vi "slow_control_2_06.vi"() -> ()   [LabVIEW 2018]
uses:
  <vilib>/DAQmx/read.llb/DAQmx Read (Analog 1D DBL NChan 1Samp).vi
  <vilib>/DAQmx/create/channels.llb/DAQmx Create Channel (AI-Voltage-Basic).vi
  <vilib>/DAQmx/create/channels.llb/DAQmx Create Channel (AI-Current-Basic).vi
  <vilib>/DAQmx/create/channels.llb/DAQmx Create Channel (AI-Temperature-RTD).vi
  <vilib>/DAQmx/miscellaneous.llb/DAQmx Fill In Error Info.vi
  <instrlib>/Lake Shore 335/Lake Shore 335.lvlib
  <instrlib>/CAEN PSM/CAEN PSM.lvlib
  <resource>/objmgr/daqmx.rc
panel:
  out "Channel Names":string[](array[string])
  out "Heater":dbl
  out "Coldhead":dbl
  out "Cycle number":i32
  in  "Cycles to execute":dbl=5.0 format="%#_13g"
  out "Moving average Det. P":dbl
  in  "N samples":i32=20
  in  "Allows tabs on \nfront panel":T1(tab)
  out "Valid example:":string
  in  "Specify which temperature sensors are\ninside the detector, separated with a comma.\nNumbers only, single commas, no empty strings!":string="10,11,12,13,14,15"
  in  "Anode ch.":enum16{"1", "2", "3", "4"}(ring)=enum."3"
  in  "CAEN unit selector":enum16{"CAEN 1", "CAEN 2"}(ring)
  in  "Multipliers":dbl[](array[numeric])=[1.0, 1.0, 1.0, 1.0, 1.0, 1.0, 1.0, 1.0]
  in  "Offsets\nsubtracted":dbl[](array[numeric])=[0.0, 0.0, 0.0, 0.0, 0.0, 0.0, 0.0, 0.0]
  in  "Channel Names (9207, ai8:15)":string[](array[string])=["i0", "i1", "i2", "i3", "i4", "i5", "i6", "i7"] caption="\"Other\""
  in  "Flow meter input:":T2(ring)=enum."v3"
  in  "Detector pressure input:":T2(ring)
  in  "Channel Names (9207, ai0:7)":string[](array[string])=["v0", "v1", "v2", "v3", "v4", "v5", "v6", "v7"] caption="\"Other\""
  in  "Multipliers":dbl[](array[numeric])=[0.2, 1.0, 1.0, 28.409091, 1.0, 1.0, 1.0, 1.0]
  in  "Offsets\nsubtracted":dbl[](array[numeric])=[0.002, 0.0, 0.0, 0.44376, 0.0, 0.0, 0.0, 0.0]
  in  "Voltage channels":tag[](array[tag])=["9207/ai0", "9207/ai1", "9207/ai2", "9207/ai3", "9207/ai4", "9207/ai5", "9207/ai6", "9207/ai7"]
  in  "COM-port CAEN 1":refnum<visa-resource-name>
  in  "COM-port CAEN 2":refnum<visa-resource-name>
  out "Temp B":dbl
  out "Temp A":dbl
  out "LakeShore readings 2":dbl[](array[numeric])
  in  "Run lakeshore?":bool
  in  "ID Query":bool=TRUE
  in  "COM-port LakeShore":refnum<visa-resource-name>
  in  "PID settings":cluster{"P":dbl, "I":dbl, "D":dbl}={"P"=50.0, "I"=20.0, "D"=120.0}
  in  "Setpoint (°C)":dbl=-100.0 format="%.1f"
  in  "Heater range":u16(ring) items=["Off", "Low (On)", "Medium", "High"]
  in  "Current channels":tag[](array[tag])=["9207/ai8", "9207/ai9", "9207/ai10", "9207/ai11", "9207/ai12", "9207/ai13", "9207/ai14", "9207/ai15"]
  in  "Channel Names (CAEN)":string[](array[string])=["PMT 1", "PMT 2", "Anode", "Cathode", "Top gate", "Bottom gate", "Other 1", "Other 2"]
  in  "RTD Type":i32(ring)=12481 items=["Pt3750"=12481, "Pt3851"=10071, "Pt3911"=12482, "Pt3916"=10069, "Pt3920"=10053, "Pt3928"=12483, "Custom"=10137]
  in  "Module 1 channels (slot 1)":tag[](array[tag])
  in  "Current Excitation Source":i32(ring)=10230 items=["Internal"=10200, "External"=10167, "None"=10230]
  in  "Resistance Configuration":i32(ring)=2 items=["2-Wire"=2, "3-Wire"=3, "4-Wire"=4]
  in  "R (T = 0°C):":dbl
  in  "B":dbl
  in  "A":dbl
  in  "C":dbl
  in  "Module 2 channels (slot 2)":tag[](array[tag])
  out "Array":i32[](array[numeric])
  out "9207 (V; A) Converted":dbl[](array[numeric])
  out "9216 #1 (°C)":dbl[](array[numeric])
  out "9216 #2 (°C)":dbl[](array[numeric])
  out "Readouts (V, mA)":dbl[](array[numeric]) format="%0.2f"
  out "Det.P input #":i32
  out "Flow input #":i32
  in  "T 20":bool
  in  "T 19":bool
  in  "T 18":bool
  in  "T 17":bool
  in  "T 16":bool
  in  "T 15":bool
  in  "Detector P":bool
  in  "Overpressure threshold":dbl
  in  "Underpressure threshold":dbl
  out "Comm. status":bool
  in  "High Temp threshold":dbl format="%#_13g"
  in  "Low Temp threshold":dbl format="%#_13g"
  in  "Ignore Initialization Errors":bool=TRUE caption="Ignore init. errors?"
  out "LakeShore status":bool
  out "NI mod1 (P) status":bool
  out "CAEN 1 status":bool
  out "CAEN 2 status":bool
  out "Initialization status":bool
  in  "Temperature channel selector":u16(ring)=10 items=["10"=10, "11"=11, "12"=12, "13"=13, "14"=14, "15"=15, "Average"=666]
  out "Heater power (%)":cluster{timestamp[], dbl[]}[](graph)
  out "Flow (SLPM)":cluster{timestamp[], dbl[]}[](graph)
  out "9207 (ai0:7)":cluster{timestamp[], dbl[]}[](graph)
  out "Phase Diagram":cluster{"X":dbl, "Y":dbl}[](graph)
  out "Temperature":cluster{timestamp[], dbl[]}[](graph)
  in  "N samples":i32=30
  out "Average Flow (SLPM)":dbl caption="Average Flow (SLPM), of"
  in  "Pause?":bool
  out "Integrated Flow (SL)":dbl
  in  "Reset?":bool
  out "LakeShore readings":dbl[](array[numeric])
  in  "Temperature Channel Selector":u16(ring) items=["10"=10, "11"=11, "12"=12, "13"=13, "14"=14, "15"=15]
  out "Historical Large Phase Diagram":cluster{dbl[], dbl[]}[](graph)
  out "Large Phase Diagram":cluster{"X":dbl, "Y":dbl}[](graph)
  in  "Temperature Channel Selector":u16(ring)=666 items=["10"=10, "11"=11, "12"=12, "13"=13, "14"=14, "15"=15, "Average"=666]
  in  "Scale.Range:Minimum 8":dbl
  in  "Scale.Range:Maximum 8":dbl=4000.0
  in  "Scale.Range:Minimum 7":dbl
  in  "Scale.Range:Maximum 7":dbl=4000.0
  in  "Scale.Range:Minimum 6":dbl=-3000.0
  in  "Scale.Range:Maximum 6":dbl
  in  "Scale.Range:Minimum 5":dbl
  in  "Scale.Range:Maximum 5":dbl=3000.0
  in  "Scale.Range:Minimum 4":dbl=-5000.0
  in  "Scale.Range:Maximum 4":dbl
  in  "Scale.Range:Maximum 3":dbl=4000.0
  in  "Scale.Range:Minimum 3":dbl
  in  "Scale.Range:Maximum 2":dbl=1000.0
  in  "Scale.Range:Minimum 2":dbl
  out "CAEN 1.1":dbl(knob) scale=0.0..1000.0
  out "CAEN 1.1":string
  in  "Scale.Range:Maximum":dbl=1000.0
  in  "Scale.Range:Minimum":dbl
  out "CAEN 2.3 2":string
  out "CAEN 2.2 2":string
  out "Channel Names":string[](array[string])
  out "CAEN 2.3":dbl(knob) scale=0.0..4000.0
  out "CAEN 2.2":dbl(knob) scale=0.0..4000.0
  out "CAEN 2.1":string
  out "CAEN 2.0":string
  out "CAEN 1.3":string
  out "CAEN 1.2":string
  out "CAEN 1.0":string
  out "Channel Names":string[](array[string])
  in  "Set to zero":bool
  out "CAEN 2.1":dbl(knob)
  out "CAEN 2.0":dbl(knob) scale=0.0..3000.0
  in  "Apply Voltage":bool
  in  "VSet (V)":dbl[](array[numeric])
  in  "IMax (uA)":dbl[](array[numeric])
  in  "VMax (V)":dbl[](array[numeric])
  out "CAEN 1.3":dbl(knob)
  out "CAEN 1.2":dbl(knob) scale=0.0..4000.0
  out "CAEN 1.0":dbl(knob) scale=0.0..1000.0
  out "Vmon (V)":dbl[](array[numeric])
  out "IMon (uA)":dbl[](array[numeric])
  in  "Read V every N cycles":i16=120
  in  "Reset anode":bool
  in  "Kill every Y minutes":i32=10
  in  "Keep off for X seconds":i32=10
  out "?":bool
  out "Killed":bool
  out "Restarted":bool
  out "Anode times":dbl[](array[numeric]) format="%_12f"
  out "Anode times 2":timestamp[](array[timestamp])
  in  "Kill voltage":bool
  in  "stop":bool
  out "Voltages":dbl[](array[numeric])
  out "Started up?":bool
  out "TOBA appended":dbl[][](array[numeric])
  in  "Read T every N cycles":i32=2
  out "Time until next cycle":dbl format="%.3g"
  in  "Time per cycle (s)":i32=2 caption="Time Target (s)"
  # "<- Proof of concept for New/Old T + New P"
  # "NI 9216 Temperature settings"
  # "CAEN settings"
  # "NI 9207 Voltage settings"
  # "If RTD type is custom,\nspecify the Callendar-\nVan Dusen parameters"
  # "Anode connected to:"
  # "Channel:"
  # "Lakeshore settings"
  # "NI 9207 Current settings"
  # "Connection settings"
  # "Gain (P) (XX.X)"
  # "Reset (I) (XX.X)"
  # "Rate (D) (X.X%)"
  # "Move to Quick Temp tab ^"
  # "Alarm indicators"
  # "Thresholds"
  # "Alarm conditions"
  # "Data"
  # "Time of last reset"
  # "Scale:"
  # "to"
  # "to"
  # "Scale:"
  # "Time of last reactivation"
  # "Settings"
  # "to"
  # "Scale:"
  # "to"
  # "Scale:"
  # "Scale:"
  # "to"
  # "Scale:"
  # "to"
  # "Scale:"
  # "to"
  # "to"
  # "Scale:"
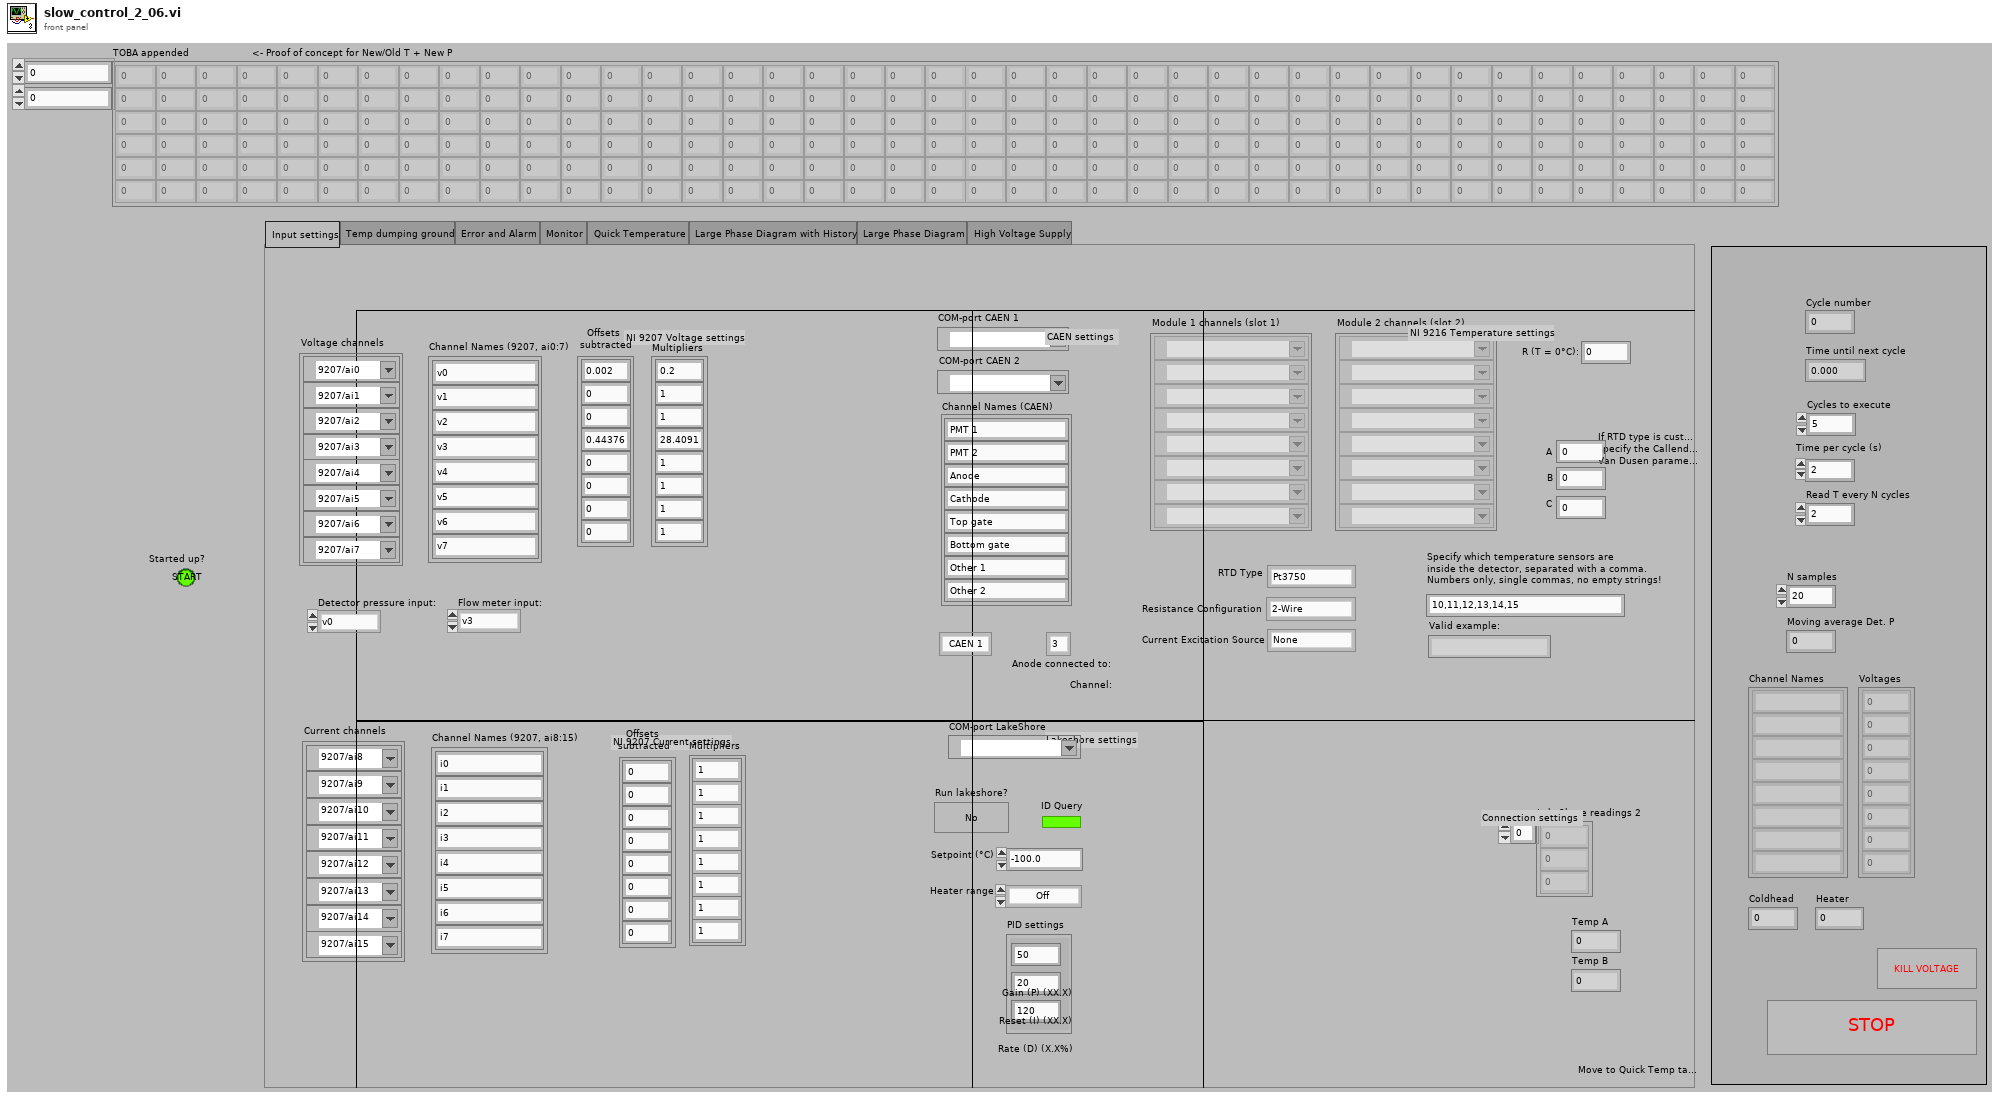
[diagram p1: front panel]
types:
  T1 = enum32{"Input settings", "Temp dumping ground", "Error and Alarm", "Monitor", "Quick Temperature", "Large Phase Diagram with History", "Large Phase Diagram", "High Voltage Supply"}
  T2 = enum16{"v0", "v1", "v2", "v3", "v4", "v5", "v6", "v7"}
  T3 = cluster{"Baud Rate":u32, "Parity":u16, "Data Bits":u16, "Stop Bits":u16, "Flow Control":u16}
  T4 = cluster{"VISA resource name out":refnum<visa-resource-name>, "error out":errorcluster}
  T5 = cluster{"task out":refnum<k21>, "error out":errorcluster}
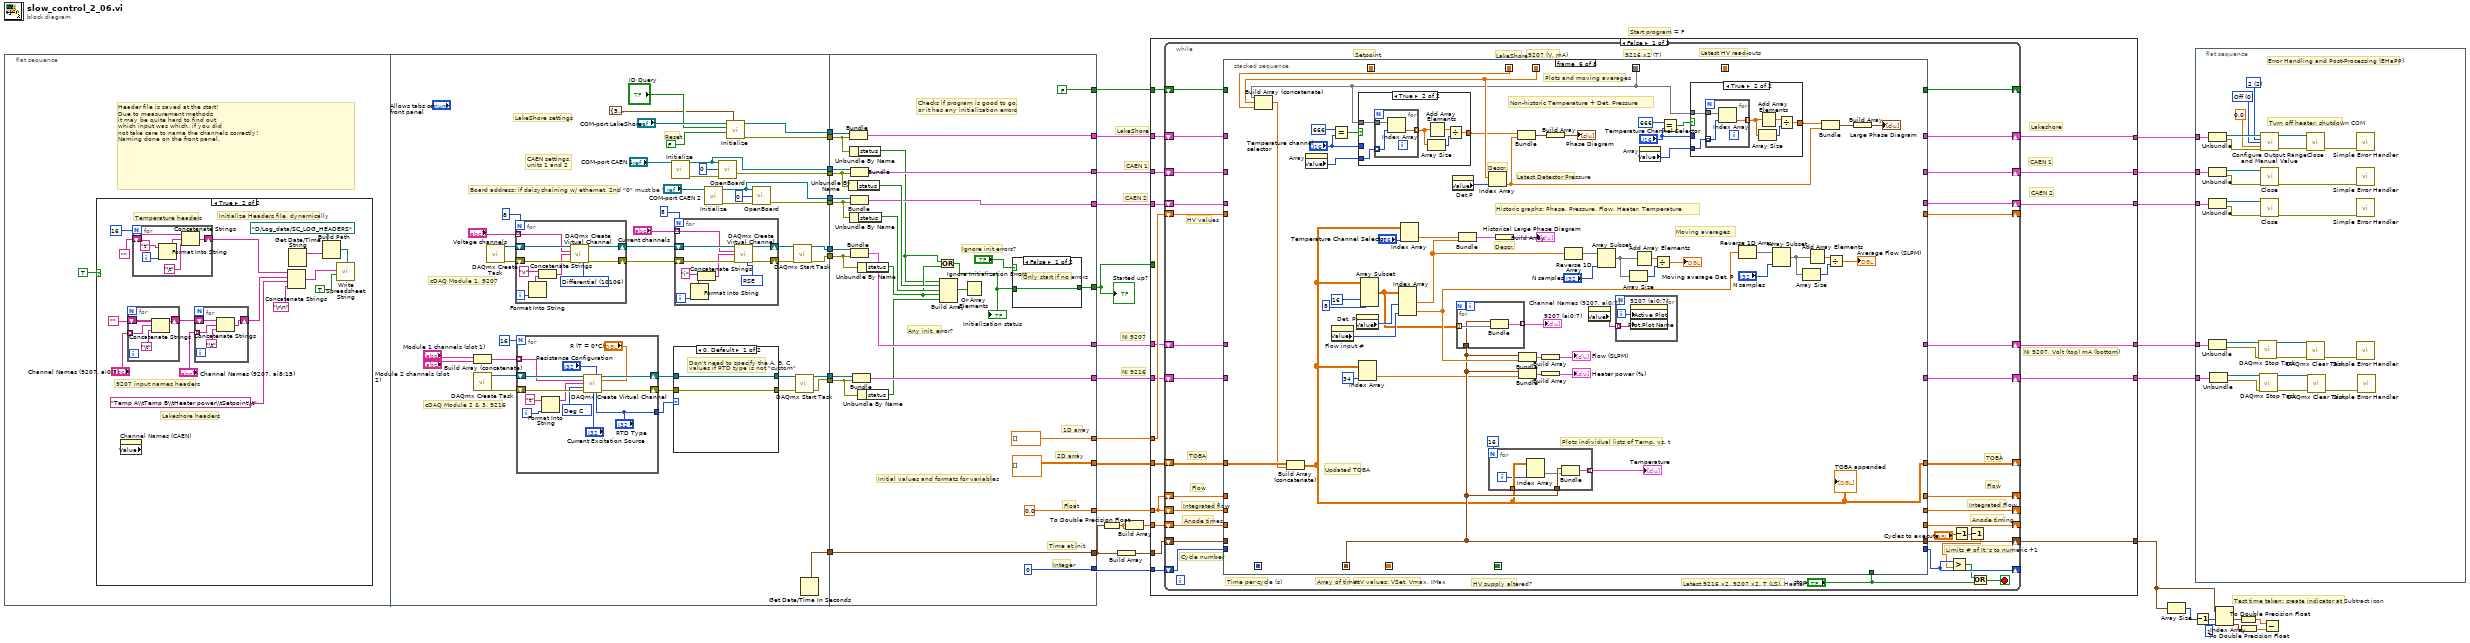
[diagram p0: block diagram]
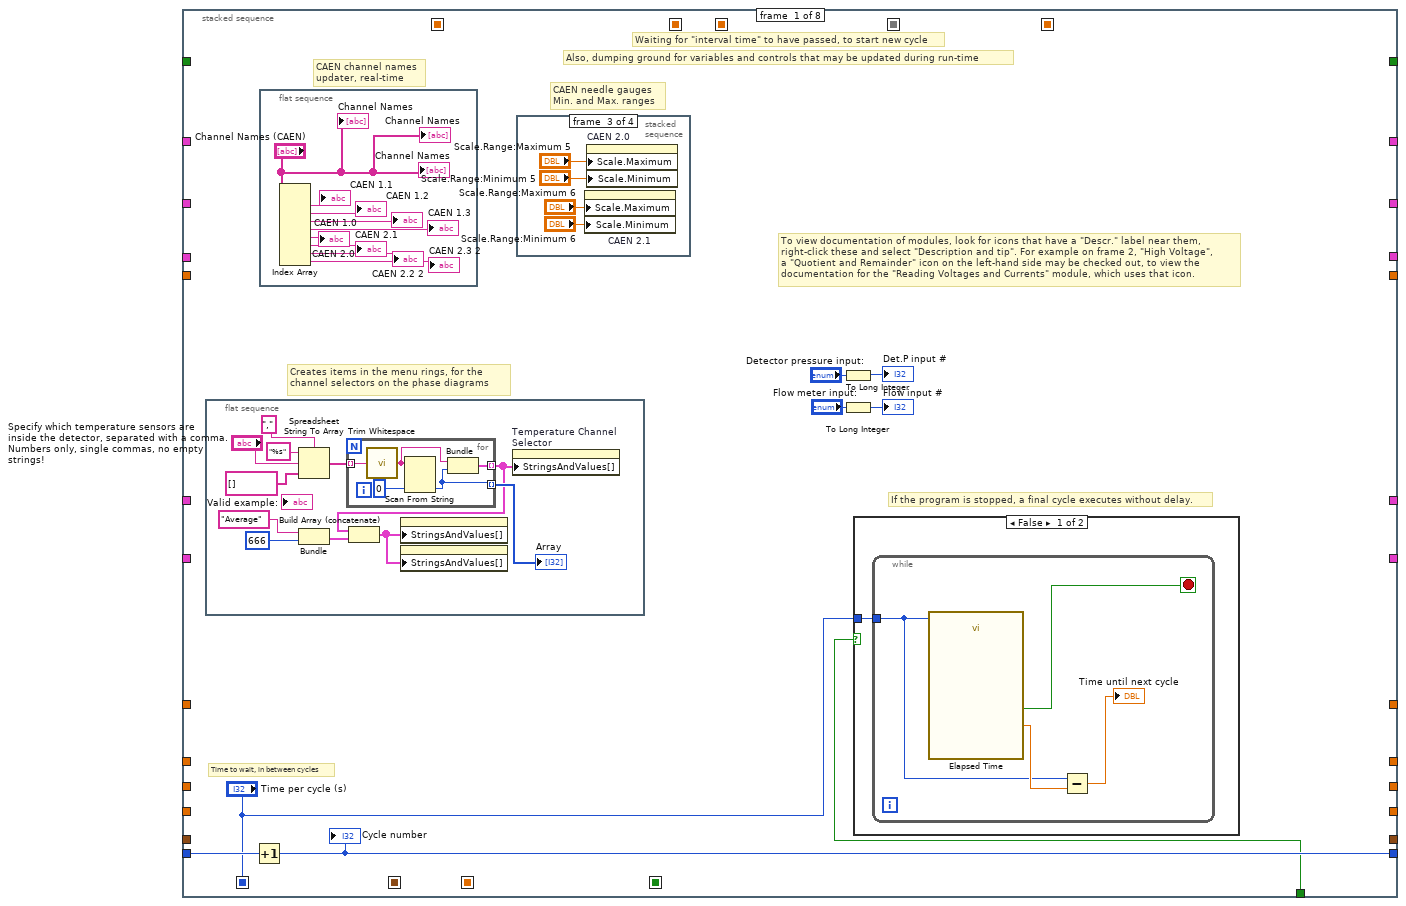
[diagram p2: hidden frame]
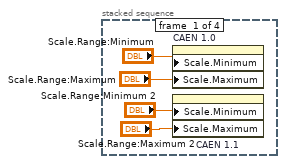
[diagram p3: hidden frame]
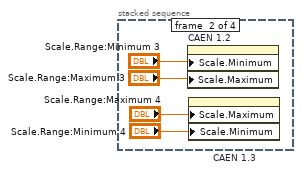
[diagram p4: hidden frame]
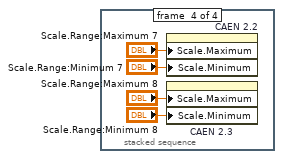
[diagram p5: hidden frame]
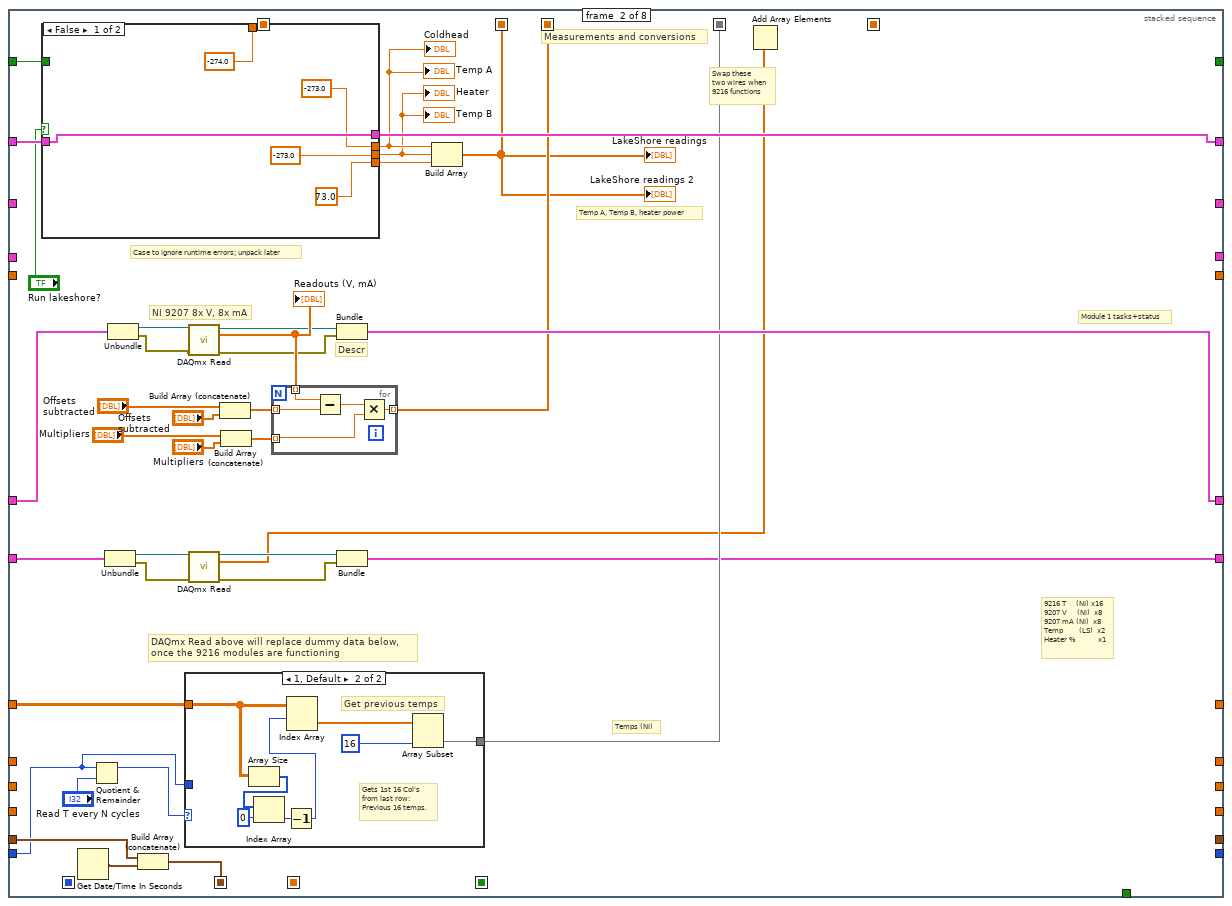
[diagram p7: hidden frame]
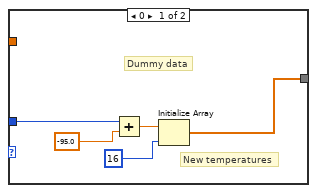
[diagram p8: hidden frame]
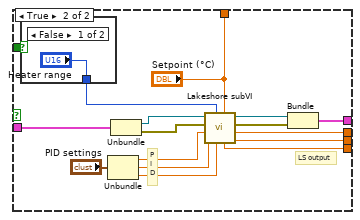
[diagram p9: hidden frame]
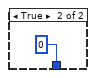
[diagram p10: hidden frame]
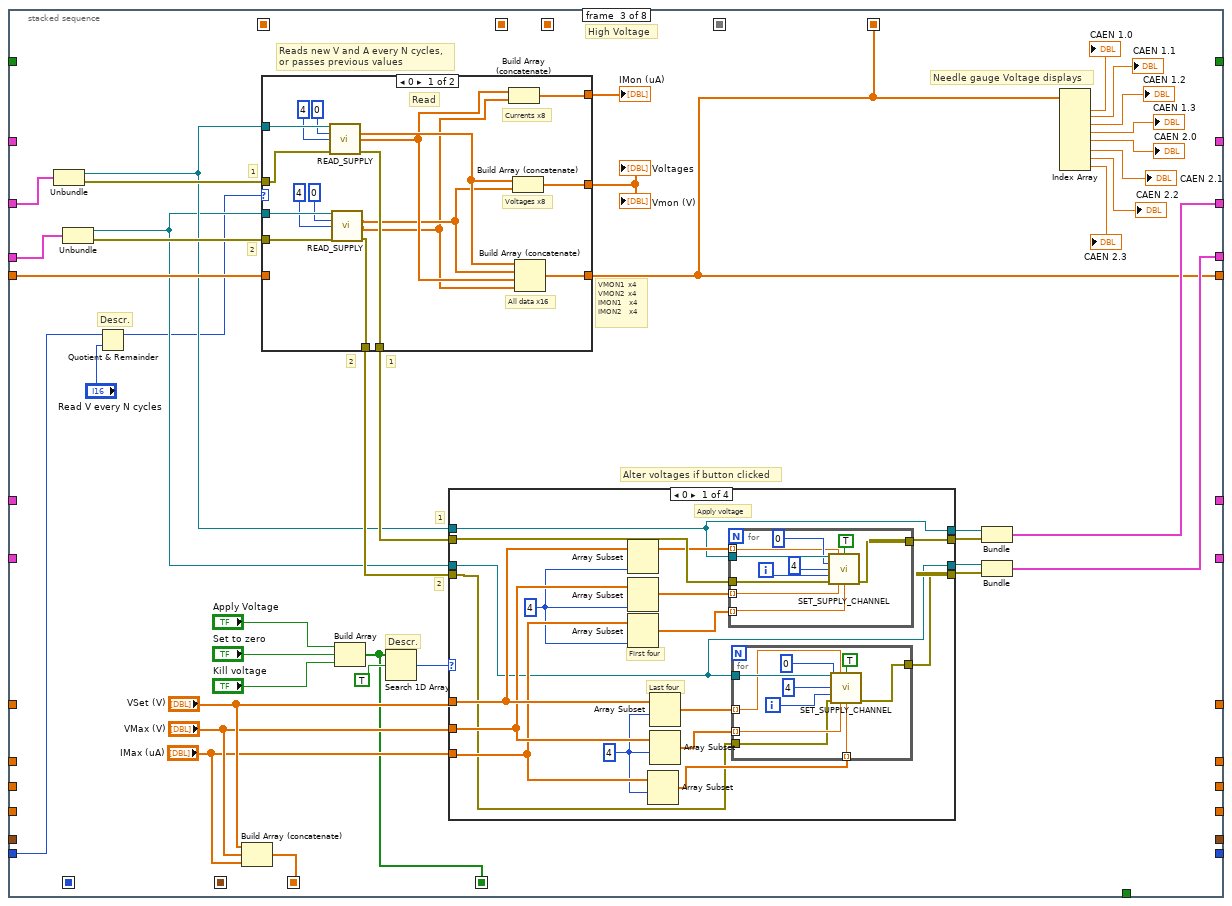
[diagram p11: hidden frame]
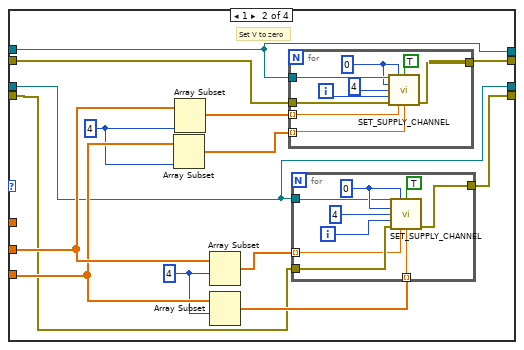
[diagram p12: hidden frame]
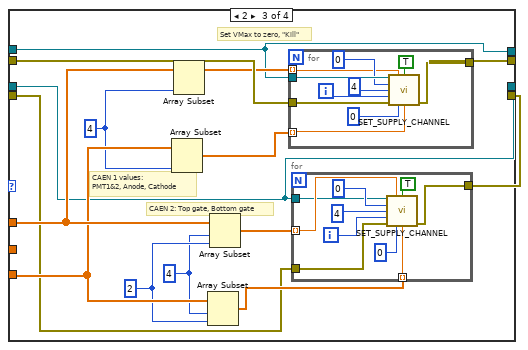
[diagram p13: hidden frame]
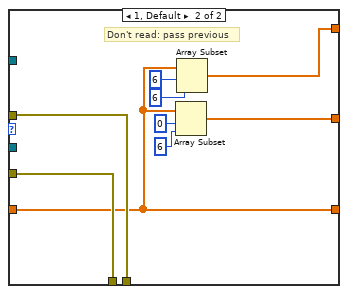
[diagram p15: hidden frame]
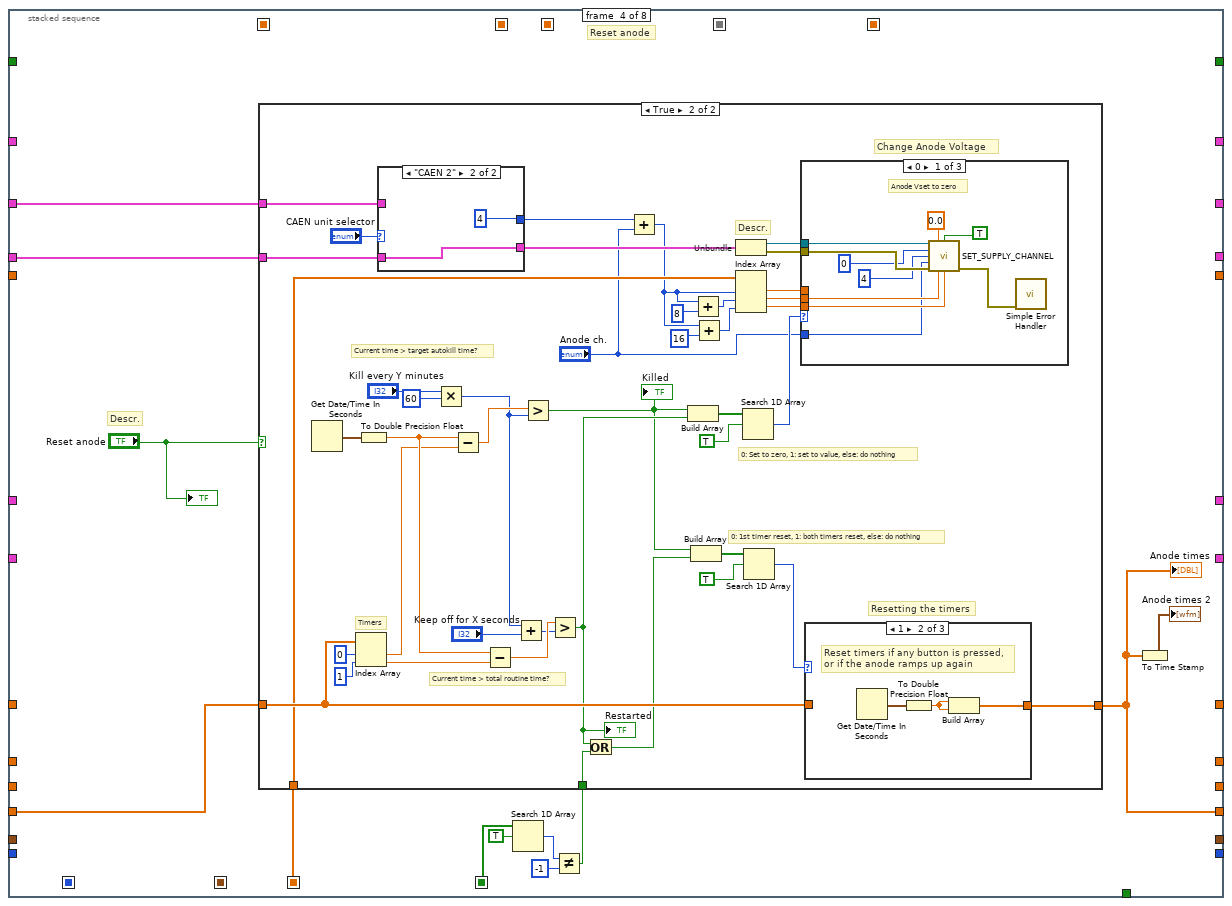
[diagram p16: hidden frame]
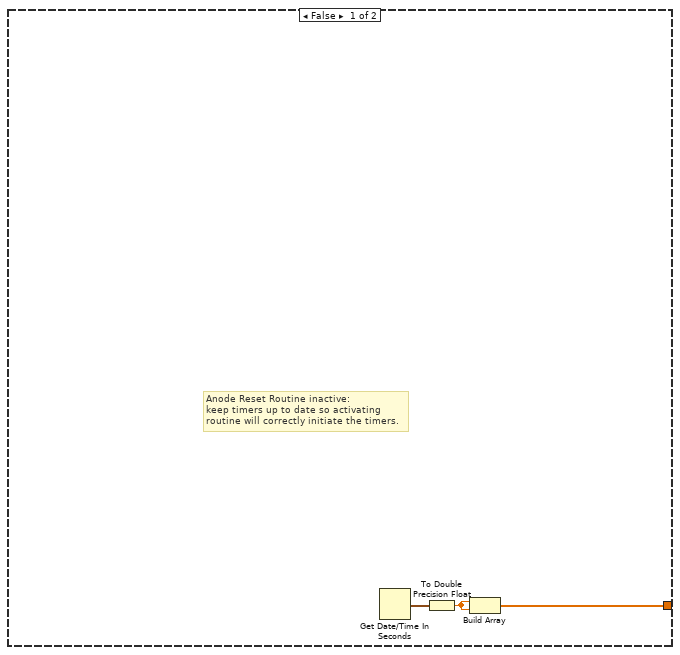
[diagram p17: hidden frame]
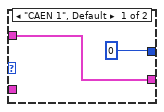
[diagram p18: hidden frame]
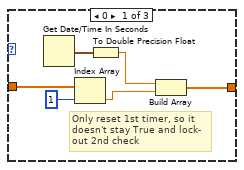
[diagram p19: hidden frame]
diagram:
  # "NI 9216"
  # "Test time taken: create indicator at Subtract icon"
  # "NI 9207"
  # "Start program = F"
  # "CAEN 2"
  # "CAEN 1"
  # "LakeShore"
  n1 = flat-sequence {
    tunnel: [w108] -> w39
    tunnel: [w107] -> w38
    tunnel: [w95] -> w37
    tunnel: [w104] -> w36
    tunnel: [w85] -> w35
    tunnel: [w103] -> w30
    tunnel: [w99] -> w22
    tunnel: [w98] -> w21
    tunnel: [w86] -> w12
    tunnel: [w80] -> w4
    tunnel: [w79] -> w3
    tunnel: w39 -> [w180]
    tunnel: w38 -> [w179]
    tunnel: w37 -> [w177]
    tunnel: w36 -> [w176]
    tunnel: w35 -> [w166]
    tunnel: [w181] -> w19
    tunnel: [0.0] -> w18
    tunnel: [dbl[] []] -> w34
    tunnel: [dbl[][] []] -> w5
    tunnel: [0] -> w33
    tunnel: [w178] -> w32
    tunnel: [w175] -> w31
    tunnel: [w174] -> w17
    tunnel: w30 -> [w174]
    tunnel: w22 -> [w172]
    tunnel: w21 -> [w171]
    tunnel: [w170] -> w20
    tunnel: [FALSE] -> w13
    tunnel: w12 -> [w167]
    tunnel: [w165] -> w11
    tunnel: w4 -> [w157]
    tunnel: w3 -> [w156]
    tunnel: [w155] -> w2
    frame #0 {
      # "Header file is saved at the start!\nDue to measurement methods\nit may be quite hard to find out\nwhich input was which, if you did\nnot take care to name the channels correctly!\nNaming done on the front panel."
      n2 = case shown="True" TRUE {
        frame False {
        }
        frame True {
          # "Lakeshore headers"
          # "9207 input names headers"
          # "Temperature headers"
          # "Initialize Headers file, dynamically"
          n3 = property on="Channel Names (CAEN)" class="Arr (strict)" props=["Value"]() -> ()  [unwired: 2 in, 3 out]
          n4 = for {
            shift-right: [w62] -> w44
            shift-left: "" -> [w63]
            tunnel: "Channel Names (9207, ai0:7)" -> [w60] mode=indexing
            n5 = Concatenate Strings(w63, w60, "\t") -> (w62:string)
          }
          n6 = for {
            N: 16 -> [_]
            shift-right: [w64] -> w47
            shift-left: "" -> [w65]
            i -> [w69]
            n7 = Format Into String(initial string="t", w69) -> (resulting string=w67:string)  [unwired: 2 in, 1 out]
            n8 = Concatenate Strings(w65, w67, "\t") -> (w64:string)
          }
          n9 = for {
            shift-right: [w57] -> w43
            shift-left: w44 -> [w59]
            tunnel: "Channel Names (9207, ai8:15)" -> [w56] mode=indexing
            n10 = Concatenate Strings(w59, w56, "\t") -> (w57:string)
          }
          n11 = Concatenate Strings(w47, w43, "Temp A\\tTemp B\\tHeater power\\tSetpoint\\t", "\r\n") -> (w46:string)
          n12 = Get Date/Time String() -> (date string=w50:string)  [unwired: 3 in, 1 out]
          n13 = Build Path(base path=path "D:/Log_data/SC_LOG_HEADERS" ("file path (dialog if empty)"), name or relative path=w50) -> (appended path=w51:path)
          n14 = call <vilib>:"Write Spreadsheet String.vi"("append to file? (new file:F)"=TRUE, "spreadsheet string"=w46, "file path (dialog if empty)"=w51) -> ()  [unwired: 7 in, 2 out]
        }
      }
    }
    frame #1 {
      # "cDAQ Module 2 & 3, 9216"
      # "cDAQ Module 1, 9207"
      # "Board address: if daisychaining w/ ethernet, 2nd \"0\" must be \"1\""
      # "CAEN settings,\nunits 1 and 2"
      # "Reset"
      # "LakeShore settings"
      n15 = call <vilib>:"DAQmx Create Task.vi"() -> ("task out"=w78:refnum<k21>, "error out"=w81:errorcluster)  [unwired: 14 in]
      n16 = Build Array (concatenate)("Module 1 channels (slot 1)", "Module 2 channels (slot 2)") -> (w75:tag[])
      n17 = call <vilib>:"DAQmx Create Task.vi"() -> ("task out"=w94:refnum<k21>, "error out"=w93:errorcluster)  [unwired: 14 in]
      n18 = for {
        N: 8 -> [_]
        shift-right: [w149] -> w90
        shift-left: w94 -> [w148]
        shift-right: [w150] -> w89
        shift-left: w93 -> [w146]
        tunnel: "Voltage channels" -> [w147] mode=indexing
        i -> [w152]
        w144 = 10106 items=["Default"=-1, "RSE"=10083, "NRSE"=10078, "Differential"=10106, "Pseudodifferential"=12529] ("input terminal configuration")
        n19 = Format Into String(w152) -> (resulting string=w151:string)  [unwired: 3 in, 1 out]
        n20 = Concatenate Strings("v" ("string"), w151) -> (w145:string)
        n21 = call-poly <vilib>:"DAQmx Create Virtual Channel.vi"("task in"=w148, "input terminal configuration"=w144, "physical channels"=w147, "name to assign"=w145, "error in"=w146) -> ("task out"=w149:refnum<k21>, "error out"=w150:errorcluster)  [unwired: 9 in]
      }
      n22 = for {
        N: 16 -> [_]
        shift-right: [w130] -> w74
        shift-left: w78 -> [w133]
        shift-right: [w131] -> w73
        shift-left: w81 -> [w132]
        tunnel: w75 -> [w129] mode=indexing
        tunnel: ["RTD Type"] -> w70
        i -> [w127]
        w124 = 10143 items=["Deg C"=10143, "Deg F"=10144, "Kelvins"=10325, "Deg R"=10145, "From Custom Scale"=10065] ("units")
        n23 = Format Into String(initial string="t", w127) -> (resulting string=w126:string)  [unwired: 2 in, 1 out]
        n24 = call-poly <vilib>:"DAQmx Create Virtual Channel.vi"("task in"=w133, "resistance configuration"="Resistance Configuration", "physical channels"=w129, "r0"="R (T = 0°C):", "name to assign"=w126, "units"=w124, "error in"=w132, "current excitation source"="Current Excitation Source", "rtd type"="RTD Type") -> ("task out"=w130:refnum<k21>, "error out"=w131:errorcluster)  [unwired: 5 in]
      }
      n25 = call <instrlib>:"Initialize.vi"("VISA resource name"="COM-port CAEN 1") -> ("error out"=w105:errorcluster, "VISA resource name out"=w95:refnum<visa-resource-name>)  [unwired: 9 in]
      n26 = case shown="0, Default" w70 {
        tunnel: w74 -> [w113 w117]
        tunnel: w73 -> [w112 w116]
        tunnel: [w113 w115] -> w72
        tunnel: [w112 w114] -> w71
        frame 0, Default {
          # "Don't need to specify the A, B, C\nvalues if RTD type is not \"custom\""
        }
        frame 10137 {
          # "RTD type =  \"custom\""
          n27 = property class="DAQmx Channel"(reference=w117, error in=w116, "AI.RTD.A"="A", "AI.RTD.B"="B", "AI.RTD.C"="C") -> (reference out=w115:refnum<k21>, error out=w114:errorcluster)
        }
      }
      n28 = for {
        N: 8 -> [_]
        shift-right: [w135] -> w87
        shift-left: w90 -> [w142]
        shift-right: [w134] -> w88
        shift-left: w89 -> [w141]
        tunnel: "Current channels" -> [w140] mode=indexing
        i -> [w139]
        w143 = 10083 items=["default"=-1, "RSE"=10083, "NRSE"=10078, "Differential"=10106, "Pseudodifferential"=12529] ("input terminal configuration")
        n29 = Format Into String(w139) -> (resulting string=w137:string)  [unwired: 3 in, 1 out]
        n30 = Concatenate Strings("i", w137) -> (w136:string)
        n31 = call-poly <vilib>:"DAQmx Create Virtual Channel.vi"("task in"=w142, "input terminal configuration"=w143, "physical channels"=w140, "name to assign"=w136, "error in"=w141) -> ("task out"=w135:refnum<k21>, "error out"=w134:errorcluster)  [unwired: 9 in]
      }
      n32 = call <instrlib>:"Initialize.vi"("VISA resource name"="COM-port CAEN 2") -> ("error out"=w100:errorcluster, "VISA resource name out"=w99:refnum<visa-resource-name>)  [unwired: 9 in]
      n33 = call <instrlib>:"OpenBoard.vi"("error in (no error)"=w105, "Board Address"=0, "VISA resource name"=w95) -> ("error out"=w104:errorcluster)  [unwired: 7 in, 1 out]
      n34 = call <instrlib>:"Initialize.vi"("Serial Configuration"=T3 {"Baud Rate"=57600, "Parity"=1, "Data Bits"=7, "Stop Bits"=10, "Flow Control"=0}, "Reset (True)"=FALSE ("Reset (LakeShore)"), "ID Query (True)"="ID Query", "VISA resource name"="COM-port LakeShore") -> ("error out"=w107:errorcluster, "VISA resource name out"=w108:refnum<visa-resource-name>)  [unwired: 6 in]
      n35 = call <instrlib>:"OpenBoard.vi"("error in (no error)"=w100, "Board Address"=u8 0, "VISA resource name"=w99) -> ("error out"=w98:errorcluster)  [unwired: 7 in, 1 out]
      n36 = call <vilib>:"DAQmx Start Task.vi"("task/channels in"=w87, "error in"=w88) -> ("task out"=w86:refnum<k21>, "error out"=w85:errorcluster)  [unwired: 12 in]
      n37 = call <vilib>:"DAQmx Start Task.vi"("task/channels in"=w72, "error in"=w71) -> ("task out"=w80:refnum<k21>, "error out"=w79:errorcluster)  [unwired: 12 in]
      n38 = Get Date/Time In Seconds() -> (seconds since 1Jan1904=w103:timestamp)
    }
    frame #2 {
      # "Initial values and formats for variables"
      # "Time at init."
      # "Integer"
      # "2D array"
      # "1D array"
      # "Float"
      # "Checks if program is good to go,\nor it has any initialization errors"
      # "Ignore init errors?"
      # "Any init. error?"
      n39 = Unbundle By Name(w176) -> ("status"=w182:bool)
      n40 = Unbundle By Name(w179) -> ("status"=w159:bool)
      n41 = Bundle("VISA resource name out"=w180, "error out"=w179) -> (w178:T4)  [unwired: 1 in]
      n42 = Unbundle By Name(w171) -> ("status"=w173:bool)
      n43 = Bundle("VISA resource name out"=w172, "error out"=w171) -> (w170:T4)  [unwired: 1 in]
      n44 = Bundle("task out"=w167, "error out"=w166) -> (w165:T5)  [unwired: 1 in]
      n45 = Bundle("VISA resource name out"=w177, "error out"=w176) -> (w175:T4)  [unwired: 1 in]
      n46 = Bundle("task out"=w157, "error out"=w156) -> (w155:T5)  [unwired: 1 in]
      n47 = Unbundle By Name(w166) -> ("status"=w160:bool)
      n48 = Unbundle By Name(w156) -> ("status"=w154:bool)
      n49 = Or(x=w159, y=w160) -> (x .or. y?=w158:bool)
      "Initialization status" <- w158
      n50 = Build Array(w159, w182, w160, w173, w154) -> (w183:bool[])
      n51 = Or Array Elements(Boolean array=w183) -> ()  [unwired: 1 out]
      n52 = case shown="False" "Ignore Initialization Errors" {
        tunnel: [w184 FALSE] -> w181
        tunnel: w158 -> [w184 _]
        frame False {
          # "Only start if no errors"
        }
        frame True {
          # "Always start program"
        }
      }
    }
  }
  n53 = To Double Precision Float(number=w17) -> (double precision float=w16:dbl)
  n54 = Build Array(w17) -> (w29:timestamp[])
  n55 = Build Array(w16, w16) -> (w15:dbl[])
  n56 = case shown="False" w19 {
    selector: w19 -> [_ w784]
    tunnel: [_ w784] -> _
    tunnel: w34 -> [w196 _]
    tunnel: w33 -> [w203 _]
    tunnel: w5 -> [w202 _]
    tunnel: w32 -> [w197 w782]
    tunnel: w31 -> [w199 w781]
    tunnel: w29 -> [w201 _]
    tunnel: [w200 timestamp[] []] -> w25
    tunnel: w20 -> [w198 w780]
    tunnel: w18 -> [w192 _]
    tunnel: w15 -> [w195 _]
    tunnel: [w194 w782] -> w14
    tunnel: w13 -> [w193 _]
    tunnel: w11 -> [w191 w779]
    tunnel: [w190 w781] -> w10
    tunnel: [w189 w780] -> w9
    tunnel: [w188 w779] -> w8
    tunnel: w2 -> [w187 w778]
    tunnel: [w186 w778] -> w1
    frame False {
      # "NI 9207, Volt (top) mA (bottom)"
      # "CAEN 2"
      # "CAEN 1"
      # "Lakeshore"
      n57 = while {
        shift-right: [w230] -> _
        shift-left: w203 -> [w235]
        shift-right: [w232] -> _
        shift-left: w202 -> [w221]
        shift-right: [w222] -> w200
        shift-left: w201 -> [w231]
        shift-right: [w224] -> w190
        shift-left: w199 -> [w216]
        shift-right: [w226] -> _
        shift-left: w196 -> [w229]
        shift-right: [w223] -> w189
        shift-left: w198 -> [w228]
        shift-right: [w225] -> w194
        shift-left: w197 -> [w227]
        shift-right: [w209] -> _
        shift-left: w192 -> [w218]
        shift-right: [w208] -> _
        shift-left: w192 -> [w219]
        shift-right: [w215] -> _
        shift-left: w195 -> [w217]
        shift-right: [w213] -> _
        shift-left: w193 -> [w214]
        shift-right: [w211] -> w188
        shift-left: w191 -> [w212]
        shift-right: [w206] -> w186
        shift-left: w187 -> [w207]
        stop <- w233 stop-if-true
        # "LakeShore"
        # "9216 x2 (T)"
        # "9207 (V, mA)"
        # "HV supply altered?"
        # "Setpoint"
        # "Anode timing"
        # "Anode times"
        # "Integrated flow"
        # "Flow"
        # "Flow"
        # "Integrated Flow"
        # "TOBA"
        # "Array of times"
        # "Latest HV read-outs"
        # "Time per cycle (s)"
        # "Cycle number"
        # "HV values: VSet, Vmax, IMax"
        # "HV values"
        # "TOBA"
        # "Latest 9216 x2, 9207 x2, T (LS), Heater% (LS)"
        # "Limits # of It.'s to numeric +1"
        n58 = stacked-sequence {
          seq-local: [_ _ w378 _ _ _ _ _] -> [_ _ _ w550 _ _ _ _]
          seq-local: ["Time per cycle (s)" _ _ _ _ _ _ _] -> [_ _ _ _ _ _ w755 _]
          seq-local: [_ _ w369 _ _ _ _ _] -> [_ _ _ _ _ _ w754 _]
          seq-local: [_ w322 _ _ _ _ _ _] -> [_ _ _ _ w640 w655 _ _]
          seq-local: [_ _ w372 _ _ _ _ _] -> [_ _ _ w553 _ _ _ _]
          seq-local: [_ w315 _ _ _ _ _ _] -> [_ _ _ _ _ _ w758 _]
          seq-local: [_ w310 _ _ _ _ _ _] -> [_ _ _ _ w633 w679 w742 _]
          seq-local: [_ w309 _ _ _ _ _ _] -> [_ _ _ _ w634 w669 w743 _]
          seq-local: [_ w297 _ _ _ _ _ _] -> [_ _ _ _ _ w677 w741 _]
          tunnel: [w242 _ _ _ _ _ _ _] -> w230
          tunnel: "stop" -> [w241 _ _ _ _ _ _ _]
          tunnel: w235 -> [w243 w311 w400 _ _ _ _ _]
          tunnel: w221 -> [_ w312 _ _ _ w681 _ _]
          tunnel: [_ _ _ _ _ w653 _ _] -> w232
          tunnel: w231 -> [_ w324 _ _ _ _ _ _]
          tunnel: w216 -> [_ _ w407 w551 _ _ _ w777]
          tunnel: w229 -> [_ _ w405 _ _ _ _ _]
          tunnel: w228 -> [_ _ w404 w542 _ _ _ w776]
          tunnel: w227 -> [_ w325 _ _ _ _ _ w775]
          tunnel: [_ w326 _ _ _ _ _ _] -> w225
          tunnel: [_ _ w369 _ _ _ _ _] -> w226
          tunnel: [_ _ w386 _ _ _ _ _] -> w224
          tunnel: [_ _ w383 _ _ _ _ _] -> w223
          tunnel: [_ _ _ _ _ w655 _ _] -> w222
          tunnel: w218 -> [_ _ _ _ w637 _ _ _]
          tunnel: w219 -> [_ _ _ _ w639 _ _ _]
          tunnel: w217 -> [_ _ _ w552 _ _ _ _]
          tunnel: [_ _ _ w546 _ _ _ _] -> w215
          tunnel: w214 -> [_ w318 _ _ _ _ _ _]
          tunnel: [_ _ _ _ _ _ _ FALSE] -> w213
          tunnel: w212 -> [_ w317 _ _ _ _ _ w773]
          tunnel: [_ w313 _ _ _ _ _ _] -> w211
          tunnel: [_ _ _ _ w636 _ _ _] -> w209
          tunnel: [_ _ _ _ w635 _ _ _] -> w208
          tunnel: w207 -> [_ w296 _ _ _ _ _ w759]
          tunnel: [_ w291 _ _ _ _ _ _] -> w206
          frame #0 {
            # "Creates items in the menu rings, for the channel selectors on the phase diagrams"
            # "Also, dumping ground for variables and controls that may be updated during run-time"
            # "CAEN needle gauges\nMin. and Max. ranges"
            # "CAEN channel names\nupdater, real-time"
            # "To view documentation of modules, look for icons that have a \"Descr.\" label near them,\nright-click these and select \"Description and tip\". For example on frame 2, \"High Voltage\",\na \"Quotient and Remainder\" icon on the left-hand side may be checked out, to view the\ndocumentation for the \"Reading Voltages and Currents\" module, which uses that icon."
            # "Time to wait, in between cycles"
            # "If the program is stopped, a final cycle executes without delay."
            # "Waiting for \"interval time\" to have passed, to start new cycle"
            n59 = flat-sequence {
              frame #0 {
                n60 = Spreadsheet String To Array(delimiter (Tab)=",", format string="%s", spreadsheet string="Specify which temperature sensors are\ninside the detector, separated with a comma.\nNumbers only, single commas, no empty strings!", array type (2D Dbl)=string[] []) -> (array=w250:string[])
                n61 = Bundle("Average", 666) -> (w247:cluster{string, i32})  [unwired: 1 in]
                n62 = for {
                  tunnel: w250 -> [w259] mode=indexing
                  tunnel: [w256] -> w244 mode=indexing
                  tunnel: [w255] -> w246 mode=indexing
                  n63 = call <vilib>:"Trim Whitespace.vi"("string"=w259) -> ("trimmed string"=w257:string)  [unwired: 1 in]
                  n64 = Scan From String(input string=w257, default 1=0) -> (output 1=w255:i32)  [unwired: 3 in, 3 out]
                  n65 = Bundle("trimmed string"=w257, w255) -> (w256:cluster{"trimmed string":string, i32})  [unwired: 1 in]
                }
                "Array" <- w246
                n66 = Build Array (concatenate)(w244, w247) -> (w245:cluster{"trimmed string":string, i32}[])
                n67 = property on="Temperature channel selector" class="Ring (strict)"("StringsAndValues[]"=w245) -> ()  [unwired: 2 in, 2 out]
                n68 = property on="Temperature Channel Selector" class="Ring (strict)"("StringsAndValues[]"=w245) -> ()  [unwired: 2 in, 2 out]
                n69 = property on="Temperature Channel Selector" class="Ring (strict)"("StringsAndValues[]"=w244) -> ()  [unwired: 2 in, 2 out]
              }
            }
            n70 = Increment(x=w243) -> (x+1=w242:i32)
            "Cycle number" <- w242
            n71 = flat-sequence {
              frame #0 {
                n72 = Index Array(array="Channel Names (CAEN)") -> (element #1=→"CAEN 1.0":string, element #2=→"CAEN 1.1":string, element #3=→"CAEN 1.2":string, element #4=→"CAEN 1.3":string, element #5=→"CAEN 2.0":string, element #6=→"CAEN 2.1":string, element #7=→"CAEN 2.2 2":string, element #8=→"CAEN 2.3 2":string)  [unwired: 8 in]
                "Channel Names" <- "Channel Names (CAEN)"
                "Channel Names" <- "Channel Names (CAEN)"
                "Channel Names" <- "Channel Names (CAEN)"
              }
            }
            n73 = stacked-sequence {
              frame #0 {
                n74 = property on="CAEN 1.0" class="Knob (strict)"("Scale.Minimum"="Scale.Range:Minimum", "Scale.Maximum"="Scale.Range:Maximum") -> ()  [unwired: 2 in, 2 out]
                n75 = property on="CAEN 1.1" class="Knob (strict)"("Scale.Minimum"="Scale.Range:Minimum 2", "Scale.Maximum"="Scale.Range:Maximum 2") -> ()  [unwired: 2 in, 2 out]
              }
              frame #1 {
                n76 = property on="CAEN 1.2" class="Knob (strict)"("Scale.Minimum"="Scale.Range:Minimum 3", "Scale.Maximum"="Scale.Range:Maximum 3") -> ()  [unwired: 2 in, 2 out]
                n77 = property on="CAEN 1.3" class="Knob (strict)"("Scale.Maximum"="Scale.Range:Maximum 4", "Scale.Minimum"="Scale.Range:Minimum 4") -> ()  [unwired: 2 in, 2 out]
              }
              frame #2 {
                n78 = property on="CAEN 2.1" class="Knob (strict)"("Scale.Maximum"="Scale.Range:Maximum 6", "Scale.Minimum"="Scale.Range:Minimum 6") -> ()  [unwired: 2 in, 2 out]
                n79 = property on="CAEN 2.0" class="Knob (strict)"("Scale.Maximum"="Scale.Range:Maximum 5", "Scale.Minimum"="Scale.Range:Minimum 5") -> ()  [unwired: 2 in, 2 out]
              }
              frame #3 {
                n80 = property on="CAEN 2.2" class="Knob (strict)"("Scale.Maximum"="Scale.Range:Maximum 7", "Scale.Minimum"="Scale.Range:Minimum 7") -> ()  [unwired: 2 in, 2 out]
                n81 = property on="CAEN 2.3" class="Knob (strict)"("Scale.Maximum"="Scale.Range:Maximum 8", "Scale.Minimum"="Scale.Range:Minimum 8") -> ()  [unwired: 2 in, 2 out]
              }
            }
            n82 = To Long Integer(number="Detector pressure input:") -> (32bit integer=→"Det.P input #":i32)
            n83 = To Long Integer(number="Flow meter input:") -> (32bit integer=→"Flow input #":i32)
            n84 = case shown="False" w241 {
              tunnel: "Time per cycle (s)" -> [w285 _]
              frame False {
                n85 = while {
                  tunnel: w285 -> [w287]
                  stop <- w289 stop-if-true
                  n86 = call "Elapsed Time"("Time Target (s)"=w287) -> ("Elapsed Time (s)"=w288:dbl, "Time has Elapsed"=w289:bool)  [unwired: 11 in, 6 out]
                  n87 = Subtract(x=w287, y=w288) -> (x-y=→"Time until next cycle":dbl)
                }
              }
              frame True {
              }
            }
          }
          frame #1 {
            # "DAQmx Read above will replace dummy data below,\nonce the 9216 modules are functioning"
            # "Swap these\ntwo wires when\n9216 functions"
            # "Descr"
            # "NI 9207 8x V, 8x mA"
            # "Case to ignore runtime errors; unpack later"
            # "Module 1 tasks+status"
            # "Temps (NI)"
            # "9216 T     (NI) x16\n9207 V     (NI)  x8\n9207 mA (NI)  x8\nTemp        (LS)  x2\nHeater %           x1"
            # "Temp A, Temp B, heater power"
            # "Measurements and conversions"
            n88 = case shown="False" "Run lakeshore?" {
              tunnel: [w349 w357] -> w326
              tunnel: w325 -> [w349 w356]
              tunnel: [-273.0 ("Input A") w355] -> w321
              tunnel: [-273.0 ("Input B") w354] -> w320
              tunnel: [73.0 ("Heater 1 (%)") w353] -> w319
              tunnel: w318 -> [_ w352]
              tunnel: [-274.0 "Setpoint (°C)"] -> w315
              frame False {
              }
              frame True {
                # "LS output"
                # "P\nI\nD"
                n89 = case shown="False" w352 {
                  tunnel: ["Heater range" 0] -> w360
                  frame False {
                  }
                  frame True {
                  }
                }
                n90 = Unbundle("PID settings") -> ("P"=w363:dbl, "I"=w362:dbl, "D"=w361:dbl)
                n91 = Unbundle(w356) -> ("VISA resource name out"=w365:refnum<visa-resource-name>, "error out"=w364:errorcluster)
                n92 = call "Lakeshore subVI.vi"("Setpoint"="Setpoint (°C)", "Rate (D) (X.X %)"=w361, "Range"=w360, "Reset (I) (XX.X)"=w362, "Gain (P) (XX.X)"=w363, "error in (no error)"=w364, "VISA resource name"=w365) -> ("Input B"=w354:dbl, "Input A"=w355:dbl, "error out"=w358:errorcluster, "VISA resource name out"=w359:refnum<visa-resource-name>, "Heater 1 (%)"=w353:dbl)
                n93 = Bundle("VISA resource name out"=w359, "error out"=w358) -> (w357:T4)  [unwired: 1 in]
              }
            }
            "Temp A" <- w321
            "Temp B" <- w320
            "Heater" <- w320
            "Coldhead" <- w321
            n94 = Get Date/Time In Seconds() -> (seconds since 1Jan1904=w323:timestamp)
            n95 = Quotient & Remainder(x=w311, y="Read T every N cycles") -> (x-y*floor(x/y)=w314:i32)  [unwired: 1 out]
            n96 = Unbundle(w296) -> ("task out"=w295:refnum<k21>, "error out"=w294:errorcluster)
            n97 = Unbundle(w317) -> ("task out"=w301:refnum<k21>, "error out"=w300:errorcluster)
            n98 = Build Array (concatenate)(w324, w323) -> (w322:timestamp[])
            n99 = case shown="1, Default" w314 {
              tunnel: w312 -> [_ w342]
              tunnel: [w335 w338] -> w309
              tunnel: w311 -> [w334 _]
              frame 0 {
                # "Dummy data"
                # "New temperatures"
                n100 = Add(x=w334, y=-95.0 ("element")) -> (x+y=w337:dbl)
                n101 = Initialize Array(w337, 16) -> (w335:dbl[])
              }
              frame 1, Default {
                # "Gets 1st 16 Col's\nfrom last row:\nPrevious 16 temps."
                # "Get previous temps"
                n102 = Array Size(array=w342) -> (size(s)=w344:i32[])
                n103 = Index Array(array=w344, index=0) -> (element=w345:i32)
                n104 = Decrement(x=w345) -> (x-1=w341:i32)
                n105 = Index Array(array=w342, index (row)=w341) -> (element=w340:dbl[])  [unwired: 1 in]
                n106 = Array Subset(array=w340, length=16) -> (w338:dbl[])  [unwired: 1 in]
              }
            }
            n107 = call-poly <vilib>:"DAQmx Read.vi"("task/channels in"=w301, "error in"=w300) -> ("task out"=w299:refnum<k21>, "data"=w308:dbl[], "error out"=w298:errorcluster)  [unwired: 11 in]
            "Readouts (V, mA)" <- w308
            n108 = call-poly <vilib>:"DAQmx Read.vi"("task/channels in"=w295, "error in"=w294) -> ("task out"=w293:refnum<k21>, "data"=w290:dbl[], "error out"=w292:errorcluster)  [unwired: 11 in]
            n109 = Build Array (concatenate)("Offsets\nsubtracted", "Offsets\nsubtracted") -> (w302:dbl[])
            n110 = Build Array (concatenate)("Multipliers", "Multipliers") -> (w305:dbl[])
            n111 = for {
              tunnel: w302 -> [w332] mode=indexing
              tunnel: w308 -> [w331] mode=indexing
              tunnel: w305 -> [w329] mode=indexing
              tunnel: [w328] -> w310 mode=indexing
              n112 = Subtract(x=w331, y=w332) -> (x-y=w330:dbl)
              n113 = Multiply(x=w330, y=w329) -> (x*y=w328:dbl)
            }
            n114 = Bundle("task out"=w299, "error out"=w298) -> (w313:T5)  [unwired: 1 in]
            n115 = Bundle("task out"=w293, "error out"=w292) -> (w291:T5)  [unwired: 1 in]
            n116 = Build Array(w321, w320, w319) -> (w297:dbl[])
            "LakeShore readings" <- w297
            "LakeShore readings 2" <- w297
            n117 = Add Array Elements(numeric array=w290) -> ()  [unwired: 1 out]
          }
          frame #2 {
            # "Alter voltages if button clicked"
            # "2"
            # "1"
            # "Descr."
            # "Descr."
            # "VMON1  x4 \nVMON2  x4\nIMON1    x4\nIMON2    x4"
            # "Needle gauge Voltage displays"
            # "1"
            # "2"
            # "1"
            # "2"
            # "Reads new V and A every N cycles,\nor passes previous values"
            # "High Voltage"
            n118 = Unbundle(w407) -> ("VISA resource name out"=w389:refnum<visa-resource-name>, "error out"=w406:errorcluster)
            n119 = Unbundle(w404) -> ("VISA resource name out"=w388:refnum<visa-resource-name>, "error out"=w403:errorcluster)
            n120 = Quotient & Remainder(x=w400, y="Read V every N cycles") -> (x-y*floor(x/y)=w373:i32)  [unwired: 1 out]
            n121 = Build Array (concatenate)("VSet (V)", "VMax (V)", "IMax (uA)") -> (w378:dbl[])
            n122 = case shown="0" w373 {
              tunnel: w389 -> [w532 _]
              tunnel: w406 -> [w531 w540]
              tunnel: w405 -> [_ w536]
              tunnel: w388 -> [w522 _]
              tunnel: w403 -> [w519 w541]
              tunnel: [w518 w541] -> w390
              tunnel: [w528 w540] -> w391
              tunnel: [w527 w536] -> w369
              tunnel: [w525 w537] -> w402
              tunnel: [w523 w533] -> w401
              frame 0 {
                # "All data x16"
                # "Voltages x8"
                # "Currents x8"
                # "Read"
                n123 = call "READ_SUPPLY.vi"("VISA resource name"=w532, "Board address"=u8 0, "NChannels"=u8 4, "error in (no error)"=w531) -> ("VMon values (V)"=w526:dbl[], "IMon values (uA)"=w524:dbl[], "error out"=w528:errorcluster)  [unwired: 9 in]
                n124 = call "READ_SUPPLY.vi"("VISA resource name"=w522, "Board address"=u8 0, "NChannels"=u8 4, "error in (no error)"=w519) -> ("VMon values (V)"=w517:dbl[], "IMon values (uA)"=w516:dbl[], "error out"=w518:errorcluster)  [unwired: 9 in]
                n125 = Build Array (concatenate)(w524, w516) -> (w523:dbl[])
                n126 = Build Array (concatenate)(w526, w517) -> (w525:dbl[])
                n127 = Build Array (concatenate)(w526, w517, w524, w516) -> (w527:dbl[])
              }
              frame 1, Default {
                # "Don't read: pass previous"
                n128 = Array Subset(array=w536, index=0, length=6) -> (w537:dbl[])
                n129 = Array Subset(array=w536, index=6, length=6) -> (w533:dbl[])
              }
            }
            "Voltages" <- w402
            "Vmon (V)" <- w402
            "IMon (uA)" <- w401
            n130 = Build Array("Apply Voltage", "Set to zero", "Kill voltage") -> (w372:bool[])
            n131 = Search 1D Array(1D array=w372, element=TRUE) -> (index of element=w392:i32)  [unwired: 1 in]
            n132 = case shown="0" w392 {
              tunnel: w391 -> [w424 w458 w491 w512]
              tunnel: w390 -> [w411 w448 w480 w514]
              tunnel: w389 -> [w420 w455 w488 w515]
              tunnel: w388 -> [w409 w446 w478 w513]
              tunnel: [w421 w456 w489 w512] -> w382
              tunnel: [w420 w455 w488 w515] -> w387
              tunnel: [w408 w445 w477 w514] -> w384
              tunnel: [w409 w446 w478 w513] -> w385
              tunnel: "VSet (V)" -> [w418 _ w486 _]
              tunnel: "VMax (V)" -> [w417 w453 _ _]
              tunnel: "IMax (uA)" -> [w416 w452 w485 _]
              frame 0 {
                w410 = 4 ("length")
                w415 = 4 ("length")
                # "Last four"
                # "First four"
                # "Apply voltage"
                n133 = Array Subset(array=w418, length=w415) -> (w423:dbl[])  [unwired: 1 in]
                n134 = Array Subset(array=w417, length=w415) -> (w422:dbl[])  [unwired: 1 in]
                n135 = Array Subset(array=w416, length=w415) -> (w419:dbl[])  [unwired: 1 in]
                n136 = Array Subset(array=w416, index=w410) -> (w412:dbl[])  [unwired: 1 in]
                n137 = Array Subset(array=w418, index=w410) -> (w414:dbl[])  [unwired: 1 in]
                n138 = Array Subset(array=w417, index=w410) -> (w413:dbl[])  [unwired: 1 in]
                n139 = for {
                  tunnel: w420 -> [w443]
                  tunnel: w424 -> [w442]
                  tunnel: w423 -> [w439] mode=indexing
                  tunnel: w422 -> [w437] mode=indexing
                  tunnel: w419 -> [w436] mode=indexing
                  tunnel: [w435] -> w421
                  i -> [w444]
                  n140 = call "SET_SUPPLY_CHANNEL.vi"("VISA resource name"=w443, "Voltage Level (0.0 V)"=w439, "Enable (OFF)"=TRUE, "Board address"=u8 0, "NChannels"=u8 4, "Channel (0)"=w444, "error in (no error)"=w442, "Voltage Max (0.0 V)"=w437, "Current Limit (0.00 uA)"=w436) -> ("error out"=w435:errorcluster)  [unwired: 6 in]
                }
                n141 = for {
                  tunnel: w409 -> [w434]
                  tunnel: w411 -> [w428]
                  tunnel: w414 -> [w433] mode=indexing
                  tunnel: w413 -> [w432] mode=indexing
                  tunnel: w412 -> [w431] mode=indexing
                  tunnel: [w427] -> w408
                  i -> [w430]
                  n142 = call "SET_SUPPLY_CHANNEL.vi"("VISA resource name"=w434, "Voltage Level (0.0 V)"=w433, "Enable (OFF)"=TRUE, "Board address"=u8 0, "NChannels"=u8 4, "Channel (0)"=w430, "error in (no error)"=w428, "Voltage Max (0.0 V)"=w432, "Current Limit (0.00 uA)"=w431) -> ("error out"=w427:errorcluster)  [unwired: 6 in]
                }
              }
              frame 1 {
                w447 = 4 ("length")
                w451 = 4 ("length")
                # "Set V to zero"
                n143 = Array Subset(array=w452, length=w451) -> (w454:dbl[])  [unwired: 1 in]
                n144 = Array Subset(array=w453, length=w451) -> (w457:dbl[])  [unwired: 1 in]
                n145 = Array Subset(array=w453, index=w447) -> (w450:dbl[])  [unwired: 1 in]
                n146 = Array Subset(array=w452, index=w447) -> (w449:dbl[])  [unwired: 1 in]
                n147 = for {
                  tunnel: w455 -> [w475]
                  tunnel: w458 -> [w474]
                  tunnel: w457 -> [w471] mode=indexing
                  tunnel: w454 -> [w470] mode=indexing
                  tunnel: [w469] -> w456
                  i -> [w476]
                  w468 = u8 0 ("Board address")
                  n148 = call "SET_SUPPLY_CHANNEL.vi"("VISA resource name"=w475, "Voltage Level (0.0 V)"=w468, "Enable (OFF)"=TRUE, "Board address"=w468, "NChannels"=u8 4, "Channel (0)"=w476, "error in (no error)"=w474, "Voltage Max (0.0 V)"=w471, "Current Limit (0.00 uA)"=w470) -> ("error out"=w469:errorcluster)  [unwired: 6 in]
                }
                n149 = for {
                  tunnel: w446 -> [w459]
                  tunnel: w448 -> [w464]
                  tunnel: w450 -> [w463] mode=indexing
                  tunnel: w449 -> [w462] mode=indexing
                  tunnel: [w460] -> w445
                  i -> [w465]
                  w467 = 0 ("length")
                  n150 = call "SET_SUPPLY_CHANNEL.vi"("VISA resource name"=w459, "Voltage Level (0.0 V)"=w467, "Enable (OFF)"=TRUE, "Board address"=w467, "NChannels"=u8 4, "Channel (0)"=w465, "error in (no error)"=w464, "Voltage Max (0.0 V)"=w463, "Current Limit (0.00 uA)"=w462) -> ("error out"=w460:errorcluster)  [unwired: 6 in]
                }
              }
              frame 2 {
                w479 = 4 ("length")
                w483 = 2 ("length")
                w484 = 4 ("length")
                # "CAEN 2: Top gate, Bottom gate"
                # "CAEN 1 values:\nPMT1&2, Anode, Cathode"
                # "Set VMax to zero, \"Kill\""
                n151 = Array Subset(array=w485, length=w484) -> (w487:dbl[])  [unwired: 1 in]
                n152 = Array Subset(array=w486, length=w484) -> (w490:dbl[])  [unwired: 1 in]
                n153 = Array Subset(array=w485, index=w479, length=w483) -> (w481:dbl[])
                n154 = Array Subset(array=w486, index=w479, length=w483) -> (w482:dbl[])
                n155 = for {
                  tunnel: w488 -> [w510]
                  tunnel: w491 -> [w509]
                  tunnel: w490 -> [w506] mode=indexing
                  tunnel: w487 -> [w504] mode=indexing
                  tunnel: [w503] -> w489
                  i -> [w511]
                  n156 = call "SET_SUPPLY_CHANNEL.vi"("VISA resource name"=w510, "Voltage Level (0.0 V)"=w506, "Enable (OFF)"=TRUE, "Board address"=u8 0, "NChannels"=u8 4, "Channel (0)"=w511, "error in (no error)"=w509, "Voltage Max (0.0 V)"=u8 0 ("Board address"), "Current Limit (0.00 uA)"=w504) -> ("error out"=w503:errorcluster)  [unwired: 6 in]
                }
                n157 = for {
                  tunnel: w478 -> [w492]
                  tunnel: w480 -> [w495]
                  tunnel: w482 -> [w498] mode=indexing
                  tunnel: w481 -> [w496] mode=indexing
                  tunnel: [w494] -> w477
                  i -> [w501]
                  n158 = call "SET_SUPPLY_CHANNEL.vi"("VISA resource name"=w492, "Voltage Level (0.0 V)"=w498, "Enable (OFF)"=TRUE, "Board address"=u8 0, "NChannels"=u8 4, "Channel (0)"=w501, "error in (no error)"=w495, "Voltage Max (0.0 V)"=0, "Current Limit (0.00 uA)"=w496) -> ("error out"=w494:errorcluster)  [unwired: 6 in]
                }
              }
              frame 3, Default {
                # "\"Executes\" if none of the three buttons have been clicked"
                # "Do nothing"
              }
            }
            n159 = Bundle("VISA resource name out"=w387, "error out"=w382) -> (w386:T4)  [unwired: 1 in]
            n160 = Bundle("VISA resource name out"=w385, "error out"=w384) -> (w383:T4)  [unwired: 1 in]
            n161 = Index Array(array=w369) -> (element #1=→"CAEN 1.0":dbl, element #2=→"CAEN 1.1":dbl, element #3=→"CAEN 1.2":dbl, element #4=→"CAEN 1.3":dbl, element #5=→"CAEN 2.0":dbl, element #6=→"CAEN 2.1":dbl, element #7=→"CAEN 2.2":dbl, element #8=→"CAEN 2.3":dbl)  [unwired: 8 in]
          }
          frame #3 {
            # "Descr."
            # "Reset anode"
            n162 = Search 1D Array(1D array=w553, element=TRUE) -> (index of element=w544:i32)  [unwired: 1 in]
            n163 = Not Equal?(x=w544, y=-1) -> (x != y?=w549:bool)
            n164 = case shown="True" "Reset anode" {
              tunnel: w552 -> [_ w587]
              tunnel: w551 -> [_ w563]
              tunnel: w550 -> [_ w568]
              tunnel: w549 -> [_ w588]
              tunnel: [w554 w569] -> w546
              tunnel: w542 -> [_ w562]
              frame False {
                # "Anode Reset Routine inactive:\nkeep timers up to date so activating\nroutine will correctly initiate the timers."
                n165 = Get Date/Time In Seconds() -> (seconds since 1Jan1904=w556:timestamp)
                n166 = To Double Precision Float(number=w556) -> (double precision float=w555:dbl)
                n167 = Build Array(w555, w555) -> (w554:dbl[])
              }
              frame True {
                # "Descr."
                # "0: 1st timer reset, 1: both timers reset, else: do nothing"
                # "Timers"
                # "0: Set to zero, 1: set to value, else: do nothing"
                # "Resetting the timers"
                # "Change Anode Voltage"
                # "Current time > total routine time?"
                # "Current time > target autokill time?"
                n168 = Get Date/Time In Seconds() -> (seconds since 1Jan1904=w597:timestamp)
                n169 = Index Array(array=w587, index #1=0 ("index"), index #2=1 ("index")) -> (element #1=w581:dbl, element #2=w583:dbl)
                n170 = To Double Precision Float(number=w597) -> (double precision float=w582:dbl)
                n171 = case shown="\"CAEN 2\"" "CAEN unit selector" {
                  tunnel: w563 -> [w600 _]
                  tunnel: w562 -> [_ w602]
                  tunnel: [w600 w602] -> w561
                  tunnel: [0 4] -> w559
                  frame "CAEN 1", Default {
                  }
                  frame "CAEN 2" {
                  }
                }
                n172 = Multiply(x="Kill every Y minutes", y=60) -> (x*y=w579:i32)
                n173 = Subtract(x=w582, y=w581) -> (x-y=w580:dbl)
                n174 = Subtract(x=w582, y=w583) -> (x-y=w571:dbl)
                n175 = Add(x=w579, y="Keep off for X seconds") -> (x+y=w570:i32)
                n176 = Greater?(x=w580, y=w579) -> (0:w573:bool)
                "Killed" <- w573
                n177 = Greater?(x=w571, y=w570) -> (0:w574:bool)
                "Restarted" <- w574
                n178 = Or(x=w574, y=w588) -> (x .or. y?=w577:bool)
                n179 = Add(x=w559, y="Anode ch.") -> (x+y=w557:i32)
                n180 = Build Array(w573, w574) -> (w590:bool[])
                n181 = Build Array(w573, w577) -> (w578:bool[])
                n182 = Add(x=w557, y=8) -> (x+y=w564:i32)
                n183 = Add(x=w557, y=16) -> (x+y=w565:i32)
                n184 = Unbundle(w561) -> ("VISA resource name out"=w595:refnum<visa-resource-name>, "error out"=w594:errorcluster)
                n185 = Index Array(array=w568, index #1=w557, index #2=w564, index #3=w565) -> (element #1=w593:dbl, element #2=w591:dbl, element #3=w592:dbl)
                n186 = Search 1D Array(1D array=w590, element=TRUE) -> (index of element=w589:i32)  [unwired: 1 in]
                n187 = Search 1D Array(1D array=w578, element=TRUE) -> (index of element=w575:i32)  [unwired: 1 in]
                n188 = case shown="0" w589 {
                  tunnel: w593 -> [_ w627 _]
                  tunnel: w591 -> [w615 w626 _]
                  tunnel: w592 -> [w617 w625 _]
                  tunnel: w595 -> [w622 w630 _]
                  tunnel: w594 -> [w621 w629 _]
                  tunnel: "Anode ch." -> [w613 w623 _]
                  frame 0 {
                    # "Anode Vset to zero"
                    n189 = call "SET_SUPPLY_CHANNEL.vi"("VISA resource name"=w622, "Voltage Level (0.0 V)"=0.0, "Enable (OFF)"=TRUE, "Board address"=u8 0, "NChannels"=u8 4, "Channel (0)"=w613, "error in (no error)"=w621, "Voltage Max (0.0 V)"=w615, "Current Limit (0.00 uA)"=w617) -> ("error out"=w616:errorcluster)  [unwired: 6 in]
                    n190 = call <vilib>:"Simple Error Handler.vi"("error in (no error)"=w616) -> ()  [unwired: 4 in, 5 out]
                  }
                  frame 1 {
                    # "Anode Vset applied"
                    n191 = call "SET_SUPPLY_CHANNEL.vi"("VISA resource name"=w630, "Voltage Level (0.0 V)"=w627, "Enable (OFF)"=TRUE, "Board address"=u8 0, "NChannels"=u8 4, "Channel (0)"=w623, "error in (no error)"=w629, "Voltage Max (0.0 V)"=w626, "Current Limit (0.00 uA)"=w625) -> ("error out"=w624:errorcluster)  [unwired: 6 in]
                    n192 = call <vilib>:"Simple Error Handler.vi"("error in (no error)"=w624) -> ()  [unwired: 4 in, 5 out]
                  }
                  frame 2, Default {
                    # "Do nothing"
                  }
                }
                n193 = case shown="1" w575 {
                  tunnel: [w603 w609 w612] -> w569
                  tunnel: w587 -> [w607 _ w612]
                  frame 0 {
                    # "Only reset 1st timer, so it\ndoesn't stay True and lock-\nout 2nd check"
                    n194 = Get Date/Time In Seconds() -> (seconds since 1Jan1904=w606:timestamp)
                    n195 = Index Array(array=w607, index=1) -> (element=w604:dbl)
                    n196 = To Double Precision Float(number=w606) -> (double precision float=w605:dbl)
                    n197 = Build Array(w605, w604) -> (w603:dbl[])
                  }
                  frame 1 {
                    # "Reset timers if any button is pressed,\nor if the anode ramps up again"
                    n198 = Get Date/Time In Seconds() -> (seconds since 1Jan1904=w611:timestamp)
                    n199 = To Double Precision Float(number=w611) -> (double precision float=w610:dbl)
                    n200 = Build Array(w610, w610) -> (w609:dbl[])
                  }
                  frame 2, Default {
                    # "Time difference grows \nlarger for now"
                  }
                }
              }
            }
            "Anode times" <- w546
            n201 = To Time Stamp(1:w546) -> (0:→"Anode times 2":timestamp[])
            "?" <- "Reset anode"
          }
          frame #4 {
            # "Displays"
            n202 = property on="Flow input #" class="DigNum (strict)"() -> ("Value"=w638:i32)  [unwired: 2 in, 2 out]
            n203 = Index Array(array=w633, index=w638) -> (element=w635:dbl)
            n204 = call "Average_flow_x_time.vi"("Array of timestamps"=w640, "Previous Flow"=w639, "Latest Flow"=w635) -> ("Volume (SL)"=w642:dbl)  [unwired: 8 in]
            n205 = case shown="False" "Reset?" {
              tunnel: [w645 0.0] -> w641
              tunnel: w637 -> [w645 _]
              frame False {
              }
              frame True {
              }
            }
            n206 = case shown="True" "Pause?" {
              tunnel: w641 -> [w649 w650]
              tunnel: w642 -> [w648 _]
              tunnel: [w647 w650] -> w636
              frame False {
                n207 = Add(x=w648, y=w649) -> (x+y=w647:dbl)
              }
              frame True {
              }
            }
            "Integrated Flow (SL)" <- w636
            "9207 (V; A) Converted" <- w633
            "9216 #1 (°C)" <- w634
            "9216 #2 (°C)" <- w634
          }
          frame #5 {
            # "Descr."
            # "Moving averages"
            # "Historic graphs: Phase, Pressure, Flow, Heater, Temperature"
            # "Non-historic Temperature + Det. Pressure"
            # "Updated TOBA"
            # "Descr."
            # "Latest Detector Pressure"
            # "Plots individual lists of Temp. vs. t"
            # "Plots and moving averages"
            n208 = Build Array (concatenate)(w669, w679, w677) -> (w678:dbl[])
            n209 = Build Array (concatenate)(w681, w678) -> (w653:dbl[][])
            "TOBA appended" <- w653
            n210 = property on="Array" class="Arr (strict)"() -> ("Value"=w668:i32[])  [unwired: 2 in, 2 out]
            n211 = property on="Flow input #" class="DigNum (strict)"() -> ("Value"=w658:i32)  [unwired: 2 in, 2 out]
            n212 = Equal?(x=666, y="Temperature channel selector") -> (x = y?=w670:bool)
            n213 = property on="Det. P:" class="Enum (strict)"() -> ("Value"=w660:T2)  [unwired: 2 in, 2 out]
            n214 = Index Array(array=w653, index (col)=34 ("disabled index (col)")) -> (element=w651:dbl[])  [unwired: 1 in]
            n215 = case shown="True" w670 {
              tunnel: w669 -> [w714 w720]
              tunnel: w668 -> [_ w719]
              tunnel: [w713 w715] -> w666
              tunnel: "Temperature channel selector" -> [w712 _]
              frame False {
                n216 = Index Array(array=w714, index=w712) -> (element=w713:dbl)
              }
              frame True {
                n217 = for {
                  tunnel: w720 -> [w723]
                  tunnel: w719 -> [w722] mode=indexing
                  tunnel: [w721] -> w716 mode=indexing
                  n218 = Index Array(array=w723, index=w722) -> (element=w721:dbl)
                }
                n219 = Array Size(array=w716) -> (size(s)=w718:i32)
                n220 = Add Array Elements(numeric array=w716) -> (sum=w717:dbl)
                n221 = Divide(x=w717, y=w718) -> (x/y=w715:dbl)
              }
            }
            n222 = Array Subset(array=w653, index (col)=16 ("index"), length (col)=8 ("length")) -> (w656:dbl[][])  [unwired: 2 in]
            n223 = Index Array(array=w656, index (col) #1=w660, index (col) #2=w658) -> (element #1=w659:dbl[], element #2=w657:dbl[])  [unwired: 2 in]
            n224 = Index Array(array=w653, index (col)="Temperature Channel Selector") -> (element=w664:dbl[])  [unwired: 1 in]
            n225 = property on="Det.P" class="DigNum (strict)"() -> ("Value"=w680:i32)  [unwired: 2 in, 2 out]
            n226 = for {
              tunnel: w656 -> [w709] mode=indexing
              tunnel: w655 -> [w708]
              tunnel: [w707] -> w654 mode=indexing
              n227 = Bundle(w708, w709) -> (w707:cluster{timestamp[], dbl[]})  [unwired: 1 in]
            }
            "9207 (ai0:7)" <- w654
            n228 = Bundle(w664, w659) -> (w699:cluster{dbl[], dbl[]})  [unwired: 1 in]
            n229 = Index Array(array=w679, index=w680) -> (element=w700:dbl)
            n230 = for {
              N: 16 -> [_]
              tunnel: w655 -> [w740]
              tunnel: [w739] -> w705 mode=indexing
              tunnel: w653 -> [w738]
              i -> [w737]
              n231 = Index Array(array=w738, index (col)=w737) -> (element=w736:dbl[])  [unwired: 1 in]
              n232 = Bundle(w740, w736) -> (w739:cluster{timestamp[], dbl[]})  [unwired: 1 in]
            }
            "Temperature" <- w705
            n233 = Build Array(w699) -> (→"Historical Large Phase Diagram":cluster{dbl[], dbl[]}[])
            n234 = Bundle(w666, w700) -> (w704:cluster{dbl, dbl})  [unwired: 1 in]
            n235 = Bundle(w655, w657) -> (w697:cluster{timestamp[], dbl[]})  [unwired: 1 in]
            n236 = Bundle(w655, w651) -> (w695:cluster{timestamp[], dbl[]})  [unwired: 1 in]
            n237 = Build Array(w697) -> (→"Flow (SLPM)":cluster{timestamp[], dbl[]}[])
            n238 = Build Array(w695) -> (→"Heater power (%)":cluster{timestamp[], dbl[]}[])
            n239 = Build Array(w704) -> (→"Phase Diagram":cluster{dbl, dbl}[])
            n240 = Reverse 1D Array(array=w659) -> (reversed array=w694:dbl[])
            n241 = property on="Channel Names (9207, ai0:7)" class="Arr (strict)"() -> ("Value"=w663:string[])  [unwired: 2 in, 2 out]
            n242 = Array Subset(array=w694, length="N samples") -> (w684:dbl[])  [unwired: 1 in]
            n243 = for {
              tunnel: w663 -> [w710] mode=indexing
              i -> [w711]
              n244 = property on="9207 (ai0:7)" class="XYGraph (strict)"("Active Plot"=w711, "Plot.Plot Name"=w710) -> ()  [unwired: 2 in, 2 out]
            }
            n245 = Array Size(array=w684) -> (size(s)=w683:i32)
            n246 = Add Array Elements(numeric array=w684) -> (sum=w693:dbl)
            n247 = property on="Array" class="Arr (strict)"() -> ("Value"=w674:i32[])  [unwired: 2 in, 2 out]
            n248 = Divide(x=w693, y=w683) -> (x/y=→"Moving average Det. P":dbl)
            n249 = Equal?(x=666, y="Temperature Channel Selector") -> (x = y?=w672:bool)
            n250 = case shown="True" w672 {
              tunnel: w669 -> [w726 w732]
              tunnel: w674 -> [_ w731]
              tunnel: [w725 w727] -> w676
              tunnel: "Temperature Channel Selector" -> [w724 _]
              frame False {
                n251 = Index Array(array=w726, index=w724) -> (element=w725:dbl)
              }
              frame True {
                n252 = for {
                  tunnel: w732 -> [w735]
                  tunnel: w731 -> [w734] mode=indexing
                  tunnel: [w733] -> w728 mode=indexing
                  n253 = Index Array(array=w735, index=w734) -> (element=w733:dbl)
                }
                n254 = Array Size(array=w728) -> (size(s)=w730:i32)
                n255 = Add Array Elements(numeric array=w728) -> (sum=w729:dbl)
                n256 = Divide(x=w729, y=w730) -> (x/y=w727:dbl)
              }
            }
            n257 = Reverse 1D Array(array=w657) -> (reversed array=w690:dbl[])
            n258 = Array Subset(array=w690, length="N samples") -> (w686:dbl[])  [unwired: 1 in]
            n259 = Array Size(array=w686) -> (size(s)=w685:i32)
            n260 = Add Array Elements(numeric array=w686) -> (sum=w689:dbl)
            n261 = Bundle(w676, w700) -> (w702:cluster{dbl, dbl})  [unwired: 1 in]
            n262 = Divide(x=w689, y=w685) -> (x/y=→"Average Flow (SLPM)":dbl)
            n263 = Build Array(w702) -> (→"Large Phase Diagram":cluster{dbl, dbl}[])
          }
          frame #6 {
            # "-----------DATA SAVED----------\nTemperatures (16),     NI 9216;\nVolts, Amps, (16),       NI 9207;\nTemperature (2),    Lakeshore;\nHeater power (1),  Lakeshore;\nSetpoint (1),           Lakeshore;\nCurrent time (s)                ---   ;\nCycle time (s)                    ---   ;"
            # "Saving data"
            n264 = Get Date/Time In Seconds() -> (seconds since 1Jan1904=w757:timestamp)
            n265 = To Double Precision Float(number=w757) -> (double precision float=w756:dbl)
            n266 = Build Array (concatenate)(w743, w742, w741, w758, w756, w755, w754) -> (w753:dbl[])
            n267 = Get Date/Time String() -> (date string=w747:string)  [unwired: 3 in, 1 out]
            n268 = Build Path(base path=path "D:/Log_data/SC_LOG", name or relative path=w747) -> (appended path=w746:path)
            n269 = Format Date/Time String() -> (date/time string=w751:string)  [unwired: 3 in]
            n270 = Array To Spreadsheet String(array=w753, 3:"%.3f" ("format string")) -> (spreadsheet string=w749:string)  [unwired: 1 in]
            n271 = Concatenate Strings(w751, "\t", w749) -> (w745:string)
            n272 = call <vilib>:"Write Spreadsheet String.vi"("append to file? (new file:F)"=TRUE, "spreadsheet string"=w745, "file path (dialog if empty)"=w746) -> ()  [unwired: 7 in, 2 out]
          }
          frame #7 {
            # "Alarm conditions (Temp)"
            # "Check alarms and UPS"
            n273 = Unbundle By Name(w759) -> ()  [unwired: 1 out]
            n274 = Unbundle By Name(w775) -> ("error out.status"=w772:bool)
            "LakeShore status" <- w772
            n275 = Unbundle By Name(w777) -> ("error out.status"=w771:bool)
            "CAEN 1 status" <- w771
            n276 = Unbundle By Name(w776) -> ("error out.status"=w770:bool)
            "CAEN 2 status" <- w770
            n277 = Unbundle By Name(w773) -> ("error out.status"=w769:bool)
            "NI mod1 (P) status" <- w769
            n278 = Build Array(w772, w771, w770, w769) -> (w768:bool[])
            n279 = Or Array Elements(Boolean array=w768) -> (logical OR=→"Comm. status":bool)
            n280 = Build Array("T 15", "T 16", "T 17", "T 18", "T 19", "T 20") -> (w760:bool[])
            n281 = for {
              tunnel: w760 -> [_] mode=indexing
            }
          }
        }
        n282 = Decrement(x="Cycles to execute") -> (x-1=w205:dbl)
        n283 = Decrement(x=w205) -> (x-1=w204:dbl)
        n284 = Greater?(x=w230, y=w204) -> (0:w210:bool)
        n285 = Or(x=w210, y="stop") -> (x .or. y?=w233:bool)
      }
    }
    frame True {
    }
  }
  n286 = Array Size(array=w25) -> (size(s)=w28:i32)
  n287 = Decrement(x=w28) -> (x-1=w27:i32)
  n288 = flat-sequence {
    tunnel: w14 -> [w813]
    tunnel: w10 -> [w804]
    tunnel: w9 -> [w801]
    tunnel: w8 -> [w796]
    tunnel: w1 -> [w785]
    frame #0 {
      w809 = u16 2 items=["1"=1, "2"=2] ("Heater Output (1:1)")
      w810 = u16 0 items=["Off", "Low (On)", "Medium", "High"] ("Range (0:Off)")
      # "Turn off heater, shutdown COM"
      # "Error Handling and Post-Processing (EHaPP)"
      n289 = Unbundle(w813) -> ("VISA resource name out"=w812:refnum<visa-resource-name>, "error out"=w811:errorcluster)
      n290 = Unbundle(w804) -> ("VISA resource name out"=w803:refnum<visa-resource-name>, "error out"=w802:errorcluster)
      n291 = Unbundle(w801) -> ("VISA resource name out"=w800:refnum<visa-resource-name>, "error out"=w799:errorcluster)
      n292 = Unbundle(w796) -> ("task out"=w794:refnum<k21>, "error out"=w792:errorcluster)
      n293 = Unbundle(w785) -> ("task out"=w789:refnum<k21>, "error out"=w787:errorcluster)
      n294 = call <vilib>:"DAQmx Stop Task.vi"("task/channels in"=w794, "error in"=w792) -> ("task out"=w793:refnum<k21>, "error out"=w791:errorcluster)  [unwired: 12 in]
      n295 = call <vilib>:"DAQmx Stop Task.vi"("task/channels in"=w789, "error in"=w787) -> ("task out"=w788:refnum<k21>, "error out"=w786:errorcluster)  [unwired: 12 in]
      n296 = call <instrlib>:"Configure Output Range and Manual Value.vi"("VISA resource name"=w812, "Heater Output (1:1)"=w809, "Range (0:Off)"=w810, "Manual Output (0.00 %)"=0.0, "error in (no error)"=w811) -> ("VISA resource name out"=w807:refnum<visa-resource-name>, "error out"=w806:errorcluster)  [unwired: 9 in]
      n297 = call <instrlib>:"Close.vi"("error in (no error)"=w802, "VISA resource name"=w803) -> ("error out"=w798:errorcluster)  [unwired: 9 in]
      n298 = call <instrlib>:"Close.vi"("error in (no error)"=w799, "VISA resource name"=w800) -> ("error out"=w797:errorcluster)  [unwired: 9 in]
      n299 = call <instrlib>:"Close.vi"("error in (no error)"=w806, "VISA resource name"=w807) -> ("error out"=w805:errorcluster)  [unwired: 9 in]
      n300 = call <vilib>:"DAQmx Clear Task.vi"("task in"=w793, "error in"=w791) -> ("error out"=w795:errorcluster)  [unwired: 13 in]
      n301 = call <vilib>:"DAQmx Clear Task.vi"("task in"=w788, "error in"=w786) -> ("error out"=w790:errorcluster)  [unwired: 13 in]
      n302 = call <vilib>:"Simple Error Handler.vi"("error in (no error)"=w805) -> ()  [unwired: 4 in, 5 out]
      n303 = call <vilib>:"Simple Error Handler.vi"("error in (no error)"=w798) -> ()  [unwired: 4 in, 5 out]
      n304 = call <vilib>:"Simple Error Handler.vi"("error in (no error)"=w797) -> ()  [unwired: 4 in, 5 out]
      n305 = call <vilib>:"Simple Error Handler.vi"("error in (no error)"=w795) -> ()  [unwired: 4 in, 5 out]
      n306 = call <vilib>:"Simple Error Handler.vi"("error in (no error)"=w790) -> ()  [unwired: 4 in, 5 out]
    }
  }
  n307 = Index Array(array=w25, index #1=w27, index #2=1 ("index")) -> (element #1=w26:timestamp, element #2=w6:timestamp)
  n308 = To Double Precision Float(number=w26) -> (double precision float=w24:dbl)
  n309 = To Double Precision Float(number=w6) -> (double precision float=w23:dbl)
  n310 = Subtract(x=w24, y=w23) -> ()  [unwired: 1 out]
  "Started up?" <- w19
